vi "DrawOutlines.vi"(8 "BuildingInfoArray":T5(array[cluster])=[{"BuildAverage"={"x"=197.5, "y"=307.5, "z"=77.5}, "BuildIndex"=1, "BuildMax"={"x"=337.0, "y"=500.0, "z"=155.0}, "BuildMin"={"x"=58.0, "y"=115.0, "z"=0.0}}, {"BuildAverage"={"x"=575.0, "y"=290.5, "z"=75.0}, "BuildIndex"=2, "BuildMax"={"x"=712.0, "y"=490.0, "z"=150.0}, "BuildMin"={"x"=438.0, "y"=91.0, "z"=0.0}}, {"BuildAverage"={"x"=-829.0, "y"=-490.5, "z"=36.5}, "BuildIndex"=3, "BuildMax"={"x"=-764.0, "y"=-308.0, "z"=73.0}, "BuildMin"={"x"=-894.0, "y"=-673.0, "z"=0.0}}, {"BuildAverage"={"x"=228.76190476190476, "y"=854.4761904761905, "z"=48.23809523809524}, "BuildIndex"=4, "BuildMax"={"x"=347.0, "y"=1250.0, "z"=108.0}, "BuildMin"={"x"=53.0, "y"=587.0, "z"=0.0}}, {"BuildAverage"={"x"=476.0, "y"=889.25, "z"=51.0}, "BuildIndex"=5, "BuildMax"={"x"=510.0, "y"=1250.0, "z"=102.0}, "BuildMin"={"x"=442.0, "y"=596.0, "z"=0.0}}, {"BuildAverage"={"x"=639.0, "y"=923.0, "z"=68.5}, "BuildIndex"=6, "BuildMax"={"x"=711.0, "y"=1250.0, "z"=137.0}, "BuildMin"={"x"=567.0, "y"=596.0, "z"=0.0}}, {"BuildAverage"={"x"=-264.0, "y"=966.0, "z"=40.0}, "BuildIndex"=7, "BuildMax"={"x"=-43.0, "y"=1043.0, "z"=80.0}, "BuildMin"={"x"=-485.0, "y"=889.0, "z"=0.0}}, {"BuildAverage"={"x"=954.0, "y"=-236.0, "z"=50.0}, "BuildIndex"=8, "BuildMax"={"x"=1086.0, "y"=-130.0, "z"=100.0}, "BuildMin"={"x"=822.0, "y"=-342.0, "z"=0.0}}, {"BuildAverage"={"x"=570.0, "y"=-884.5, "z"=52.0}, "BuildIndex"=9, "BuildMax"={"x"=707.0, "y"=-750.0, "z"=104.0}, "BuildMin"={"x"=433.0, "y"=-1019.0, "z"=0.0}}, {"BuildAverage"={"x"=207.0, "y"=-887.0, "z"=44.0}, "BuildIndex"=10, "BuildMax"={"x"=356.0, "y"=-755.0, "z"=88.0}, "BuildMin"={"x"=58.0, "y"=-1019.0, "z"=0.0}}, {"BuildAverage"={"x"=-154.0, "y"=-887.0, "z"=35.0}, "BuildIndex"=11, "BuildMax"={"x"=-48.0, "y"=-755.0, "z"=70.0}, "BuildMin"={"x"=-260.0, "y"=-1019.0, "z"=0.0}}, {"BuildAverage"={"x"=-380.0, "y"=-887.0, "z"=36.0}, "BuildIndex"=12, "BuildMax"={"x"=-279.0, "y"=-755.0, "z"=72.0}, "BuildMin"={"x"=-481.0, "y"=-1019.0, "z"=0.0}}, {"BuildAverage"={"x"=-1061.2, "y"=-363.6, "z"=46.5}, "BuildIndex"=13, "BuildMax"={"x"=-966.0, "y"=-106.0, "z"=93.0}, "BuildMin"={"x"=-1139.0, "y"=-683.0, "z"=0.0}}, {"BuildAverage"={"x"=-1050.75, "y"=305.0, "z"=84.0}, "BuildIndex"=14, "BuildMax"={"x"=-885.0, "y"=490.0, "z"=168.0}, "BuildMin"={"x"=-1250.0, "y"=120.0, "z"=0.0}}, {"BuildAverage"={"x"=-654.0, "y"=1031.5, "z"=42.5}, "BuildIndex"=15, "BuildMax"={"x"=-577.0, "y"=1481.0, "z"=85.0}, "BuildMin"={"x"=-731.0, "y"=582.0, "z"=0.0}}, {"BuildAverage"={"x"=969.0, "y"=-711.5, "z"=37.5}, "BuildIndex"=16, "BuildMax"={"x"=1106.0, "y"=-404.0, "z"=75.0}, "BuildMin"={"x"=832.0, "y"=-1019.0, "z"=0.0}}, {"BuildAverage"={"x"=1139.5, "y"=425.75, "z"=79.5}, "BuildIndex"=17, "BuildMax"={"x"=1452.0, "y"=1058.0, "z"=159.0}, "BuildMin"={"x"=827.0, "y"=130.0, "z"=0.0}}, {"BuildAverage"={"x"=-1017.6666666666666, "y"=1054.3333333333333, "z"=39.0}, "BuildIndex"=18, "BuildMax"={"x"=-774.0, "y"=1635.0, "z"=78.0}, "BuildMin"={"x"=-1337.0, "y"=663.0, "z"=0.0}}, {"BuildAverage"={"x"=1262.25, "y"=-572.0, "z"=52.5}, "BuildIndex"=19, "BuildMax"={"x"=1404.0, "y"=-125.0, "z"=105.0}, "BuildMin"={"x"=1183.0, "y"=-1019.0, "z"=0.0}}, {"BuildAverage"={"x"=1596.5, "y"=-168.0, "z"=60.0}, "BuildIndex"=20, "BuildMax"={"x"=1885.0, "y"=-115.0, "z"=120.0}, "BuildMin"={"x"=1308.0, "y"=-221.0, "z"=0.0}}, {"BuildAverage"={"x"=1425.0, "y"=-392.0, "z"=50.0}, "BuildIndex"=21, "BuildMax"={"x"=1461.0, "y"=-274.0, "z"=100.0}, "BuildMin"={"x"=1389.0, "y"=-510.0, "z"=0.0}}, {"BuildAverage"={"x"=1577.0, "y"=-479.0, "z"=160.0}, "BuildIndex"=22, "BuildMax"={"x"=1625.0, "y"=-438.0, "z"=320.0}, "BuildMin"={"x"=1529.0, "y"=-520.0, "z"=0.0}}, {"BuildAverage"={"x"=1577.0, "y"=-608.0, "z"=160.0}, "BuildIndex"=23, "BuildMax"={"x"=1625.0, "y"=-543.0, "z"=320.0}, "BuildMin"={"x"=1529.0, "y"=-673.0, "z"=0.0}}, {"BuildAverage"={"x"=1705.75, "y"=-342.75, "z"=37.5}, "BuildIndex"=24, "BuildMax"={"x"=1803.0, "y"=-255.0, "z"=75.0}, "BuildMin"={"x"=1558.0, "y"=-423.0, "z"=0.0}}, {"BuildAverage"={"x"=1790.167058823529, "y"=186.08470588235298, "z"=42.23529411764706}, "BuildIndex"=25, "BuildMax"={"x"=2375.0, "y"=307.69, "z"=95.0}, "BuildMin"={"x"=1548.1, "y"=86.54, "z"=0.0}}, {"BuildAverage"={"x"=-1037.0499999999997, "y"=-832.2999999999997, "z"=33.75}, "BuildIndex"=26, "BuildMax"={"x"=-949.55, "y"=-754.8, "z"=67.5}, "BuildMin"={"x"=-1139.55, "y"=-864.8, "z"=0.0}}, {"BuildAverage"={"x"=-1262.0499999999997, "y"=-923.5333333333334, "z"=35.0}, "BuildIndex"=27, "BuildMax"={"x"=-1097.05, "y"=-769.2, "z"=70.0}, "BuildMin"={"x"=-1492.05, "y"=-1039.2, "z"=0.0}}, {"BuildAverage"={"x"=-160.5, "y"=-1294.95, "z"=45.0}, "BuildIndex"=28, "BuildMax"={"x"=-53.0, "y"=-1099.95, "z"=90.0}, "BuildMin"={"x"=-268.0, "y"=-1489.95, "z"=0.0}}, {"BuildAverage"={"x"=-384.25, "y"=-1294.95, "z"=43.75}, "BuildIndex"=29, "BuildMax"={"x"=-284.25, "y"=-1099.95, "z"=87.5}, "BuildMin"={"x"=-484.25, "y"=-1489.95, "z"=0.0}}, {"BuildAverage"={"x"=-789.25, "y"=-1288.0, "z"=45.0}, "BuildIndex"=30, "BuildMax"={"x"=-576.75, "y"=-1098.0, "z"=90.0}, "BuildMin"={"x"=-1001.75, "y"=-1478.0, "z"=0.0}}, {"BuildAverage"={"x"=-1293.2, "y"=-1283.0, "z"=50.0}, "BuildIndex"=31, "BuildMax"={"x"=-1098.2, "y"=-1098.0, "z"=100.0}, "BuildMin"={"x"=-1488.2, "y"=-1468.0, "z"=0.0}}, {"BuildAverage"={"x"=-940.8500000000001, "y"=-979.9799999999998, "z"=35.0}, "BuildIndex"=32, "BuildMax"={"x"=-884.6, "y"=-940.73, "z"=70.0}, "BuildMin"={"x"=-997.1, "y"=-1019.23, "z"=0.0}}, {"BuildAverage"={"x"=-743.1111111111111, "y"=-891.7777777777778, "z"=31.11111111111111}, "BuildIndex"=33, "BuildMax"={"x"=-567.0, "y"=-755.0, "z"=70.0}, "BuildMin"={"x"=-884.0, "y"=-1019.0, "z"=0.0}}, {"BuildAverage"={"x"=133.0, "y"=-1294.95, "z"=38.75}, "BuildIndex"=34, "BuildMax"={"x"=213.0, "y"=-1099.95, "z"=77.5}, "BuildMin"={"x"=53.0, "y"=-1489.95, "z"=0.0}}, {"BuildAverage"={"x"=298.05, "y"=-1294.95, "z"=42.5}, "BuildIndex"=35, "BuildMax"={"x"=360.55, "y"=-1099.95, "z"=85.0}, "BuildMin"={"x"=235.55, "y"=-1489.95, "z"=0.0}}, {"BuildAverage"={"x"=568.25, "y"=-1294.95, "z"=41.25}, "BuildIndex"=36, "BuildMax"={"x"=718.25, "y"=-1099.95, "z"=82.5}, "BuildMin"={"x"=418.25, "y"=-1489.95, "z"=0.0}}, {"BuildAverage"={"x"=899.3999999999999, "y"=-1294.95, "z"=50.0}, "BuildIndex"=37, "BuildMax"={"x"=971.9, "y"=-1099.95, "z"=100.0}, "BuildMin"={"x"=826.9, "y"=-1489.95, "z"=0.0}}, {"BuildAverage"={"x"=1061.25, "y"=-1294.95, "z"=35.0}, "BuildIndex"=38, "BuildMax"={"x"=1130.0, "y"=-1099.95, "z"=70.0}, "BuildMin"={"x"=1000.0, "y"=-1489.95, "z"=0.0}}, {"BuildAverage"={"x"=-264.0, "y"=389.5, "z"=44.0}, "BuildIndex"=39, "BuildMax"={"x"=-38.0, "y"=500.0, "z"=88.0}, "BuildMin"={"x"=-490.0, "y"=279.0, "z"=0.0}}, {"BuildAverage"={"x"=-418.5, "y"=-226.5, "z"=37.5}, "BuildIndex"=40, "BuildMax"={"x"=-361.0, "y"=-135.0, "z"=75.0}, "BuildMin"={"x"=-476.0, "y"=-318.0, "z"=0.0}}, {"BuildAverage"={"x"=-185.5, "y"=-221.5, "z"=158.5}, "BuildIndex"=41, "BuildMax"={"x"=-58.0, "y"=-135.0, "z"=245.0}, "BuildMin"={"x"=-313.0, "y"=-308.0, "z"=0.0}}, {"BuildAverage"={"x"=394.0, "y"=-224.0, "z"=57.5}, "BuildIndex"=42, "BuildMax"={"x"=721.0, "y"=-130.0, "z"=115.0}, "BuildMin"={"x"=67.0, "y"=-318.0, "z"=0.0}}, {"BuildAverage"={"x"=-387.0, "y"=-519.5, "z"=34.0}, "BuildIndex"=43, "BuildMax"={"x"=-293.0, "y"=-356.0, "z"=68.0}, "BuildMin"={"x"=-481.0, "y"=-683.0, "z"=0.0}}, {"BuildAverage"={"x"=-154.0, "y"=-514.5, "z"=45.0}, "BuildIndex"=44, "BuildMax"={"x"=-48.0, "y"=-356.0, "z"=90.0}, "BuildMin"={"x"=-260.0, "y"=-673.0, "z"=0.0}}, {"BuildAverage"={"x"=370.5, "y"=-513.5, "z"=42.0}, "BuildIndex"=45, "BuildMax"={"x"=712.0, "y"=-404.0, "z"=84.0}, "BuildMin"={"x"=58.0, "y"=-668.0, "z"=0.0}}, {"BuildAverage"={"x"=353.5, "y"=-464.0, "z"=60.0}, "BuildIndex"=46, "BuildMax"={"x"=534.0, "y"=-404.0, "z"=120.0}, "BuildMin"={"x"=173.0, "y"=-524.0, "z"=0.0}}, {"BuildAverage"={"x"=-634.5, "y"=-394.0, "z"=60.0}, "BuildIndex"=47, "BuildMax"={"x"=-567.0, "y"=-115.0, "z"=120.0}, "BuildMin"={"x"=-702.0, "y"=-673.0, "z"=0.0}}, {"BuildAverage"={"x"=-675.5, "y"=288.5, "z"=64.0}, "BuildIndex"=48, "BuildMax"={"x"=-572.0, "y"=495.0, "z"=128.0}, "BuildMin"={"x"=-779.0, "y"=82.0, "z"=0.0}}, {"BuildAverage"={"x"=-829.5, "y"=-197.5, "z"=62.5}, "BuildIndex"=49, "BuildMax"={"x"=-760.0, "y"=-106.0, "z"=125.0}, "BuildMin"={"x"=-899.0, "y"=-289.0, "z"=0.0}}, {"BuildAverage"={"x"=-269.25, "y"=690.0, "z"=0.0}, "BuildIndex"=50, "BuildMax"={"x"=-38.0, "y"=798.0, "z"=0.0}, "BuildMin"={"x"=-500.0, "y"=587.0, "z"=0.0}}, {"BuildAverage"={"x"=-317.25, "y"=168.5, "z"=93.75}, "BuildIndex"=51, "BuildMax"={"x"=-48.0, "y"=250.0, "z"=265.0}, "BuildMin"={"x"=-490.0, "y"=87.0, "z"=0.0}}], 11 "FloorplanArray":T6(array[cluster])=[{"xVert"=337.0, "yVert"=115.0, "zVert"=30.0, "xNorm"=0.0, "yNorm"=0.0, "zNorm"=-1.0, "BuildIndex"=1}, {"xVert"=337.0, "yVert"=115.0, "zVert"=0.0, "xNorm"=0.0, "yNorm"=0.0, "zNorm"=-1.0, "BuildIndex"=1}, {"xVert"=58.0, "yVert"=115.0, "zVert"=0.0, "xNorm"=0.0, "yNorm"=0.0, "zNorm"=-1.0, "BuildIndex"=1}, {"xVert"=58.0, "yVert"=500.0, "zVert"=0.0, "xNorm"=0.0, "yNorm"=0.0, "zNorm"=-1.0, "BuildIndex"=1}, {"xVert"=337.0, "yVert"=500.0, "zVert"=0.0, "xNorm"=0.0, "yNorm"=0.0, "zNorm"=-1.0, "BuildIndex"=1}, {"xVert"=337.0, "yVert"=115.0, "zVert"=0.0, "xNorm"=0.0, "yNorm"=0.0, "zNorm"=-1.0, "BuildIndex"=1}, {"xVert"=337.0, "yVert"=115.0, "zVert"=30.0, "xNorm"=0.0, "yNorm"=0.0, "zNorm"=-1.0, "BuildIndex"=1}, {"xVert"=712.0, "yVert"=91.0, "zVert"=30.0, "xNorm"=0.0, "yNorm"=0.0, "zNorm"=-1.0, "BuildIndex"=2}, {"xVert"=712.0, "yVert"=91.0, "zVert"=0.0, "xNorm"=0.0, "yNorm"=0.0, "zNorm"=-1.0, "BuildIndex"=2}, {"xVert"=438.0, "yVert"=91.0, "zVert"=0.0, "xNorm"=0.0, "yNorm"=0.0, "zNorm"=-1.0, "BuildIndex"=2}, {"xVert"=438.0, "yVert"=490.0, "zVert"=0.0, "xNorm"=0.0, "yNorm"=0.0, "zNorm"=-1.0, "BuildIndex"=2}, {"xVert"=712.0, "yVert"=490.0, "zVert"=0.0, "xNorm"=0.0, "yNorm"=0.0, "zNorm"=-1.0, "BuildIndex"=2}, {"xVert"=712.0, "yVert"=91.0, "zVert"=0.0, "xNorm"=0.0, "yNorm"=0.0, "zNorm"=-1.0, "BuildIndex"=2}, {"xVert"=712.0, "yVert"=91.0, "zVert"=30.0, "xNorm"=0.0, "yNorm"=0.0, "zNorm"=-1.0, "BuildIndex"=2}, {"xVert"=-764.0, "yVert"=-308.0, "zVert"=30.0, "xNorm"=0.0, "yNorm"=0.0, "zNorm"=-1.0, "BuildIndex"=3}, {"xVert"=-764.0, "yVert"=-308.0, "zVert"=0.0, "xNorm"=0.0, "yNorm"=0.0, "zNorm"=-1.0, "BuildIndex"=3}, {"xVert"=-764.0, "yVert"=-673.0, "zVert"=0.0, "xNorm"=0.0, "yNorm"=0.0, "zNorm"=-1.0, "BuildIndex"=3}, {"xVert"=-894.0, "yVert"=-673.0, "zVert"=0.0, "xNorm"=0.0, "yNorm"=0.0, "zNorm"=-1.0, "BuildIndex"=3}, {"xVert"=-894.0, "yVert"=-308.0, "zVert"=0.0, "xNorm"=0.0, "yNorm"=0.0, "zNorm"=-1.0, "BuildIndex"=3}, {"xVert"=-764.0, "yVert"=-308.0, "zVert"=0.0, "xNorm"=0.0, "yNorm"=0.0, "zNorm"=-1.0, "BuildIndex"=3}, {"xVert"=-764.0, "yVert"=-308.0, "zVert"=30.0, "xNorm"=0.0, "yNorm"=0.0, "zNorm"=-1.0, "BuildIndex"=3}, {"xVert"=53.0, "yVert"=587.0, "zVert"=30.0, "xNorm"=0.0, "yNorm"=0.0, "zNorm"=-1.0, "BuildIndex"=4}, {"xVert"=53.0, "yVert"=587.0, "zVert"=0.0, "xNorm"=0.0, "yNorm"=0.0, "zNorm"=-1.0, "BuildIndex"=4}, {"xVert"=53.0, "yVert"=1250.0, "zVert"=0.0, "xNorm"=0.0, "yNorm"=0.0, "zNorm"=-1.0, "BuildIndex"=4}, {"xVert"=216.0, "yVert"=1250.0, "zVert"=0.0, "xNorm"=0.0, "yNorm"=0.0, "zNorm"=-1.0, "BuildIndex"=4}, {"xVert"=216.0, "yVert"=654.0, "zVert"=0.0, "xNorm"=0.0, "yNorm"=0.0, "zNorm"=-1.0, "BuildIndex"=4}, {"xVert"=260.0, "yVert"=654.0, "zVert"=0.0, "xNorm"=0.0, "yNorm"=0.0, "zNorm"=-1.0, "BuildIndex"=4}, {"xVert"=260.0, "yVert"=596.0, "zVert"=0.0, "xNorm"=0.0, "yNorm"=0.0, "zNorm"=-1.0, "BuildIndex"=4}, {"xVert"=260.0, "yVert"=587.0, "zVert"=0.0, "xNorm"=0.0, "yNorm"=0.0, "zNorm"=-1.0, "BuildIndex"=4}, {"xVert"=260.0, "yVert"=596.0, "zVert"=0.0, "xNorm"=0.0, "yNorm"=0.0, "zNorm"=-1.0, "BuildIndex"=4}, {"xVert"=260.0, "yVert"=654.0, "zVert"=0.0, "xNorm"=0.0, "yNorm"=0.0, "zNorm"=-1.0, "BuildIndex"=4}, {"xVert"=260.0, "yVert"=1250.0, "zVert"=0.0, "xNorm"=0.0, "yNorm"=0.0, "zNorm"=-1.0, "BuildIndex"=4}, {"xVert"=347.0, "yVert"=1250.0, "zVert"=0.0, "xNorm"=0.0, "yNorm"=0.0, "zNorm"=-1.0, "BuildIndex"=4}, {"xVert"=347.0, "yVert"=596.0, "zVert"=0.0, "xNorm"=0.0, "yNorm"=0.0, "zNorm"=-1.0, "BuildIndex"=4}, {"xVert"=53.0, "yVert"=587.0, "zVert"=0.0, "xNorm"=0.0, "yNorm"=0.0, "zNorm"=-1.0, "BuildIndex"=4}, {"xVert"=53.0, "yVert"=587.0, "zVert"=30.0, "xNorm"=0.0, "yNorm"=0.0, "zNorm"=-1.0, "BuildIndex"=4}, {"xVert"=442.0, "yVert"=596.0, "zVert"=30.0, "xNorm"=0.0, "yNorm"=0.0, "zNorm"=-1.0, "BuildIndex"=5}, {"xVert"=442.0, "yVert"=596.0, "zVert"=0.0, "xNorm"=0.0, "yNorm"=0.0, "zNorm"=-1.0, "BuildIndex"=5}, {"xVert"=442.0, "yVert"=1250.0, "zVert"=0.0, "xNorm"=0.0, "yNorm"=0.0, "zNorm"=-1.0, "BuildIndex"=5}, {"xVert"=510.0, "yVert"=1115.0, "zVert"=0.0, "xNorm"=0.0, "yNorm"=0.0, "zNorm"=-1.0, "BuildIndex"=5}, {"xVert"=510.0, "yVert"=596.0, "zVert"=0.0, "xNorm"=0.0, "yNorm"=0.0, "zNorm"=-1.0, "BuildIndex"=5}, {"xVert"=442.0, "yVert"=596.0, "zVert"=0.0, "xNorm"=0.0, "yNorm"=0.0, "zNorm"=-1.0, "BuildIndex"=5}, {"xVert"=442.0, "yVert"=596.0, "zVert"=30.0, "xNorm"=0.0, "yNorm"=0.0, "zNorm"=-1.0, "BuildIndex"=5}, {"xVert"=711.0, "yVert"=596.0, "zVert"=30.0, "xNorm"=0.0, "yNorm"=0.0, "zNorm"=-1.0, "BuildIndex"=6}, {"xVert"=711.0, "yVert"=596.0, "zVert"=0.0, "xNorm"=0.0, "yNorm"=0.0, "zNorm"=-1.0, "BuildIndex"=6}, {"xVert"=567.0, "yVert"=596.0, "zVert"=0.0, "xNorm"=0.0, "yNorm"=0.0, "zNorm"=-1.0, "BuildIndex"=6}, {"xVert"=567.0, "yVert"=1250.0, "zVert"=0.0, "xNorm"=0.0, "yNorm"=0.0, "zNorm"=-1.0, "BuildIndex"=6}, {"xVert"=711.0, "yVert"=1250.0, "zVert"=0.0, "xNorm"=0.0, "yNorm"=0.0, "zNorm"=-1.0, "BuildIndex"=6}, {"xVert"=711.0, "yVert"=596.0, "zVert"=0.0, "xNorm"=0.0, "yNorm"=0.0, "zNorm"=-1.0, "BuildIndex"=6}, {"xVert"=711.0, "yVert"=596.0, "zVert"=30.0, "xNorm"=0.0, "yNorm"=0.0, "zNorm"=-1.0, "BuildIndex"=6}, {"xVert"=-43.0, "yVert"=889.0, "zVert"=30.0, "xNorm"=0.0, "yNorm"=0.0, "zNorm"=-1.0, "BuildIndex"=7}, {"xVert"=-43.0, "yVert"=889.0, "zVert"=0.0, "xNorm"=0.0, "yNorm"=0.0, "zNorm"=-1.0, "BuildIndex"=7}, {"xVert"=-485.0, "yVert"=889.0, "zVert"=0.0, "xNorm"=0.0, "yNorm"=0.0, "zNorm"=-1.0, "BuildIndex"=7}, {"xVert"=-485.0, "yVert"=1043.0, "zVert"=0.0, "xNorm"=0.0, "yNorm"=0.0, "zNorm"=-1.0, "BuildIndex"=7}, {"xVert"=-43.0, "yVert"=1043.0, "zVert"=0.0, "xNorm"=0.0, "yNorm"=0.0, "zNorm"=-1.0, "BuildIndex"=7}, {"xVert"=-43.0, "yVert"=889.0, "zVert"=0.0, "xNorm"=0.0, "yNorm"=0.0, "zNorm"=-1.0, "BuildIndex"=7}, {"xVert"=-43.0, "yVert"=889.0, "zVert"=30.0, "xNorm"=0.0, "yNorm"=0.0, "zNorm"=-1.0, "BuildIndex"=7}, {"xVert"=822.0, "yVert"=-130.0, "zVert"=30.0, "xNorm"=0.0, "yNorm"=0.0, "zNorm"=-1.0, "BuildIndex"=8}, {"xVert"=822.0, "yVert"=-130.0, "zVert"=0.0, "xNorm"=0.0, "yNorm"=0.0, "zNorm"=-1.0, "BuildIndex"=8}, {"xVert"=1086.0, "yVert"=-130.0, "zVert"=0.0, "xNorm"=0.0, "yNorm"=0.0, "zNorm"=-1.0, "BuildIndex"=8}, {"xVert"=1086.0, "yVert"=-342.0, "zVert"=0.0, "xNorm"=0.0, "yNorm"=0.0, "zNorm"=-1.0, "BuildIndex"=8}, {"xVert"=822.0, "yVert"=-342.0, "zVert"=0.0, "xNorm"=0.0, "yNorm"=0.0, "zNorm"=-1.0, "BuildIndex"=8}, {"xVert"=822.0, "yVert"=-130.0, "zVert"=0.0, "xNorm"=0.0, "yNorm"=0.0, "zNorm"=-1.0, "BuildIndex"=8}, {"xVert"=822.0, "yVert"=-130.0, "zVert"=30.0, "xNorm"=0.0, "yNorm"=0.0, "zNorm"=-1.0, "BuildIndex"=8}, {"xVert"=433.0, "yVert"=-750.0, "zVert"=30.0, "xNorm"=0.0, "yNorm"=0.0, "zNorm"=-1.0, "BuildIndex"=9}, {"xVert"=433.0, "yVert"=-750.0, "zVert"=0.0, "xNorm"=0.0, "yNorm"=0.0, "zNorm"=-1.0, "BuildIndex"=9}, {"xVert"=707.0, "yVert"=-750.0, "zVert"=0.0, "xNorm"=0.0, "yNorm"=0.0, "zNorm"=-1.0, "BuildIndex"=9}, {"xVert"=707.0, "yVert"=-1019.0, "zVert"=0.0, "xNorm"=0.0, "yNorm"=0.0, "zNorm"=-1.0, "BuildIndex"=9}, {"xVert"=433.0, "yVert"=-1019.0, "zVert"=0.0, "xNorm"=0.0, "yNorm"=0.0, "zNorm"=-1.0, "BuildIndex"=9}, {"xVert"=433.0, "yVert"=-750.0, "zVert"=0.0, "xNorm"=0.0, "yNorm"=0.0, "zNorm"=-1.0, "BuildIndex"=9}, {"xVert"=433.0, "yVert"=-750.0, "zVert"=30.0, "xNorm"=0.0, "yNorm"=0.0, "zNorm"=-1.0, "BuildIndex"=9}, {"xVert"=58.0, "yVert"=-755.0, "zVert"=30.0, "xNorm"=0.0, "yNorm"=0.0, "zNorm"=-1.0, "BuildIndex"=10}, {"xVert"=58.0, "yVert"=-755.0, "zVert"=0.0, "xNorm"=0.0, "yNorm"=0.0, "zNorm"=-1.0, "BuildIndex"=10}, {"xVert"=356.0, "yVert"=-755.0, "zVert"=0.0, "xNorm"=0.0, "yNorm"=0.0, "zNorm"=-1.0, "BuildIndex"=10}, {"xVert"=356.0, "yVert"=-1019.0, "zVert"=0.0, "xNorm"=0.0, "yNorm"=0.0, "zNorm"=-1.0, "BuildIndex"=10}, {"xVert"=58.0, "yVert"=-1019.0, "zVert"=0.0, "xNorm"=0.0, "yNorm"=0.0, "zNorm"=-1.0, "BuildIndex"=10}, {"xVert"=58.0, "yVert"=-755.0, "zVert"=0.0, "xNorm"=0.0, "yNorm"=0.0, "zNorm"=-1.0, "BuildIndex"=10}, {"xVert"=58.0, "yVert"=-755.0, "zVert"=30.0, "xNorm"=0.0, "yNorm"=0.0, "zNorm"=-1.0, "BuildIndex"=10}, {"xVert"=-260.0, "yVert"=-755.0, "zVert"=30.0, "xNorm"=0.0, "yNorm"=0.0, "zNorm"=-1.0, "BuildIndex"=11}, {"xVert"=-260.0, "yVert"=-755.0, "zVert"=0.0, "xNorm"=0.0, "yNorm"=0.0, "zNorm"=-1.0, "BuildIndex"=11}, {"xVert"=-48.0, "yVert"=-755.0, "zVert"=0.0, "xNorm"=0.0, "yNorm"=0.0, "zNorm"=-1.0, "BuildIndex"=11}, {"xVert"=-48.0, "yVert"=-1019.0, "zVert"=0.0, "xNorm"=0.0, "yNorm"=0.0, "zNorm"=-1.0, "BuildIndex"=11}, {"xVert"=-260.0, "yVert"=-1019.0, "zVert"=0.0, "xNorm"=0.0, "yNorm"=0.0, "zNorm"=-1.0, "BuildIndex"=11}, {"xVert"=-260.0, "yVert"=-755.0, "zVert"=0.0, "xNorm"=0.0, "yNorm"=0.0, "zNorm"=-1.0, "BuildIndex"=11}, {"xVert"=-260.0, "yVert"=-755.0, "zVert"=30.0, "xNorm"=0.0, "yNorm"=0.0, "zNorm"=-1.0, "BuildIndex"=11}, {"xVert"=-481.0, "yVert"=-755.0, "zVert"=30.0, "xNorm"=0.0, "yNorm"=0.0, "zNorm"=-1.0, "BuildIndex"=12}, {"xVert"=-481.0, "yVert"=-755.0, "zVert"=0.0, "xNorm"=0.0, "yNorm"=0.0, "zNorm"=-1.0, "BuildIndex"=12}, {"xVert"=-279.0, "yVert"=-755.0, "zVert"=0.0, "xNorm"=0.0, "yNorm"=0.0, "zNorm"=-1.0, "BuildIndex"=12}, {"xVert"=-279.0, "yVert"=-1019.0, "zVert"=0.0, "xNorm"=0.0, "yNorm"=0.0, "zNorm"=-1.0, "BuildIndex"=12}, {"xVert"=-481.0, "yVert"=-1019.0, "zVert"=0.0, "xNorm"=0.0, "yNorm"=0.0, "zNorm"=-1.0, "BuildIndex"=12}, {"xVert"=-481.0, "yVert"=-755.0, "zVert"=0.0, "xNorm"=0.0, "yNorm"=0.0, "zNorm"=-1.0, "BuildIndex"=12}, {"xVert"=-481.0, "yVert"=-755.0, "zVert"=30.0, "xNorm"=0.0, "yNorm"=0.0, "zNorm"=-1.0, "BuildIndex"=12}, {"xVert"=-1139.0, "yVert"=-240.0, "zVert"=30.0, "xNorm"=0.0, "yNorm"=0.0, "zNorm"=-1.0, "BuildIndex"=13}, {"xVert"=-1139.0, "yVert"=-240.0, "zVert"=0.0, "xNorm"=0.0, "yNorm"=0.0, "zNorm"=-1.0, "BuildIndex"=13}, {"xVert"=-1139.0, "yVert"=-106.0, "zVert"=0.0, "xNorm"=0.0, "yNorm"=0.0, "zNorm"=-1.0, "BuildIndex"=13}, {"xVert"=-966.0, "yVert"=-106.0, "zVert"=0.0, "xNorm"=0.0, "yNorm"=0.0, "zNorm"=-1.0, "BuildIndex"=13}, {"xVert"=-966.0, "yVert"=-683.0, "zVert"=0.0, "xNorm"=0.0, "yNorm"=0.0, "zNorm"=-1.0, "BuildIndex"=13}, {"xVert"=-1096.0, "yVert"=-683.0, "zVert"=0.0, "xNorm"=0.0, "yNorm"=0.0, "zNorm"=-1.0, "BuildIndex"=13}, {"xVert"=-1139.0, "yVert"=-240.0, "zVert"=0.0, "xNorm"=0.0, "yNorm"=0.0, "zNorm"=-1.0, "BuildIndex"=13}, {"xVert"=-1139.0, "yVert"=-240.0, "zVert"=30.0, "xNorm"=0.0, "yNorm"=0.0, "zNorm"=-1.0, "BuildIndex"=13}, {"xVert"=-885.0, "yVert"=490.0, "zVert"=30.0, "xNorm"=0.0, "yNorm"=0.0, "zNorm"=-1.0, "BuildIndex"=14}, {"xVert"=-885.0, "yVert"=490.0, "zVert"=0.0, "xNorm"=0.0, "yNorm"=0.0, "zNorm"=-1.0, "BuildIndex"=14}, {"xVert"=-885.0, "yVert"=120.0, "zVert"=0.0, "xNorm"=0.0, "yNorm"=0.0, "zNorm"=-1.0, "BuildIndex"=14}, {"xVert"=-1183.0, "yVert"=120.0, "zVert"=0.0, "xNorm"=0.0, "yNorm"=0.0, "zNorm"=-1.0, "BuildIndex"=14}, {"xVert"=-1250.0, "yVert"=490.0, "zVert"=0.0, "xNorm"=0.0, "yNorm"=0.0, "zNorm"=-1.0, "BuildIndex"=14}, {"xVert"=-885.0, "yVert"=490.0, "zVert"=0.0, "xNorm"=0.0, "yNorm"=0.0, "zNorm"=-1.0, "BuildIndex"=14}, {"xVert"=-885.0, "yVert"=490.0, "zVert"=30.0, "xNorm"=0.0, "yNorm"=0.0, "zNorm"=-1.0, "BuildIndex"=14}, {"xVert"=-577.0, "yVert"=1481.0, "zVert"=30.0, "xNorm"=0.0, "yNorm"=0.0, "zNorm"=-1.0, "BuildIndex"=15}, {"xVert"=-577.0, "yVert"=1481.0, "zVert"=0.0, "xNorm"=0.0, "yNorm"=0.0, "zNorm"=-1.0, "BuildIndex"=15}, {"xVert"=-577.0, "yVert"=582.0, "zVert"=0.0, "xNorm"=0.0, "yNorm"=0.0, "zNorm"=-1.0, "BuildIndex"=15}, {"xVert"=-731.0, "yVert"=582.0, "zVert"=0.0, "xNorm"=0.0, "yNorm"=0.0, "zNorm"=-1.0, "BuildIndex"=15}, {"xVert"=-731.0, "yVert"=1481.0, "zVert"=0.0, "xNorm"=0.0, "yNorm"=0.0, "zNorm"=-1.0, "BuildIndex"=15}, {"xVert"=-577.0, "yVert"=1481.0, "zVert"=0.0, "xNorm"=0.0, "yNorm"=0.0, "zNorm"=-1.0, "BuildIndex"=15}, {"xVert"=-577.0, "yVert"=1481.0, "zVert"=30.0, "xNorm"=0.0, "yNorm"=0.0, "zNorm"=-1.0, "BuildIndex"=15}, {"xVert"=832.0, "yVert"=-404.0, "zVert"=30.0, "xNorm"=0.0, "yNorm"=0.0, "zNorm"=-1.0, "BuildIndex"=16}, {"xVert"=832.0, "yVert"=-404.0, "zVert"=0.0, "xNorm"=0.0, "yNorm"=0.0, "zNorm"=-1.0, "BuildIndex"=16}, {"xVert"=1106.0, "yVert"=-404.0, "zVert"=0.0, "xNorm"=0.0, "yNorm"=0.0, "zNorm"=-1.0, "BuildIndex"=16}, {"xVert"=1106.0, "yVert"=-1019.0, "zVert"=0.0, "xNorm"=0.0, "yNorm"=0.0, "zNorm"=-1.0, "BuildIndex"=16}, {"xVert"=832.0, "yVert"=-1019.0, "zVert"=0.0, "xNorm"=0.0, "yNorm"=0.0, "zNorm"=-1.0, "BuildIndex"=16}, {"xVert"=832.0, "yVert"=-404.0, "zVert"=0.0, "xNorm"=0.0, "yNorm"=0.0, "zNorm"=-1.0, "BuildIndex"=16}, {"xVert"=832.0, "yVert"=-404.0, "zVert"=30.0, "xNorm"=0.0, "yNorm"=0.0, "zNorm"=-1.0, "BuildIndex"=16}, {"xVert"=1452.0, "yVert"=385.0, "zVert"=30.0, "xNorm"=0.0, "yNorm"=0.0, "zNorm"=-1.0, "BuildIndex"=17}, {"xVert"=1452.0, "yVert"=385.0, "zVert"=0.0, "xNorm"=0.0, "yNorm"=0.0, "zNorm"=-1.0, "BuildIndex"=17}, {"xVert"=1452.0, "yVert"=130.0, "zVert"=0.0, "xNorm"=0.0, "yNorm"=0.0, "zNorm"=-1.0, "BuildIndex"=17}, {"xVert"=827.0, "yVert"=130.0, "zVert"=0.0, "xNorm"=0.0, "yNorm"=0.0, "zNorm"=-1.0, "BuildIndex"=17}, {"xVert"=827.0, "yVert"=1058.0, "zVert"=0.0, "xNorm"=0.0, "yNorm"=0.0, "zNorm"=-1.0, "BuildIndex"=17}, {"xVert"=1452.0, "yVert"=385.0, "zVert"=0.0, "xNorm"=0.0, "yNorm"=0.0, "zNorm"=-1.0, "BuildIndex"=17}, {"xVert"=1452.0, "yVert"=385.0, "zVert"=30.0, "xNorm"=0.0, "yNorm"=0.0, "zNorm"=-1.0, "BuildIndex"=17}, {"xVert"=-1337.0, "yVert"=663.0, "zVert"=30.0, "xNorm"=0.0, "yNorm"=0.0, "zNorm"=-1.0, "BuildIndex"=18}, {"xVert"=-1337.0, "yVert"=663.0, "zVert"=0.0, "xNorm"=0.0, "yNorm"=0.0, "zNorm"=-1.0, "BuildIndex"=18}, {"xVert"=-1337.0, "yVert"=865.0, "zVert"=0.0, "xNorm"=0.0, "yNorm"=0.0, "zNorm"=-1.0, "BuildIndex"=18}, {"xVert"=-942.0, "yVert"=865.0, "zVert"=0.0, "xNorm"=0.0, "yNorm"=0.0, "zNorm"=-1.0, "BuildIndex"=18}, {"xVert"=-942.0, "yVert"=1635.0, "zVert"=0.0, "xNorm"=0.0, "yNorm"=0.0, "zNorm"=-1.0, "BuildIndex"=18}, {"xVert"=-774.0, "yVert"=1635.0, "zVert"=0.0, "xNorm"=0.0, "yNorm"=0.0, "zNorm"=-1.0, "BuildIndex"=18}, {"xVert"=-774.0, "yVert"=663.0, "zVert"=0.0, "xNorm"=0.0, "yNorm"=0.0, "zNorm"=-1.0, "BuildIndex"=18}, {"xVert"=-1337.0, "yVert"=663.0, "zVert"=0.0, "xNorm"=0.0, "yNorm"=0.0, "zNorm"=-1.0, "BuildIndex"=18}, {"xVert"=-1337.0, "yVert"=663.0, "zVert"=30.0, "xNorm"=0.0, "yNorm"=0.0, "zNorm"=-1.0, "BuildIndex"=18}, {"xVert"=1183.0, "yVert"=-1019.0, "zVert"=30.0, "xNorm"=0.0, "yNorm"=0.0, "zNorm"=-1.0, "BuildIndex"=19}, {"xVert"=1183.0, "yVert"=-1019.0, "zVert"=0.0, "xNorm"=0.0, "yNorm"=0.0, "zNorm"=-1.0, "BuildIndex"=19}, {"xVert"=1183.0, "yVert"=-125.0, "zVert"=0.0, "xNorm"=0.0, "yNorm"=0.0, "zNorm"=-1.0, "BuildIndex"=19}, {"xVert"=1279.0, "yVert"=-125.0, "zVert"=0.0, "xNorm"=0.0, "yNorm"=0.0, "zNorm"=-1.0, "BuildIndex"=19}, {"xVert"=1404.0, "yVert"=-1019.0, "zVert"=0.0, "xNorm"=0.0, "yNorm"=0.0, "zNorm"=-1.0, "BuildIndex"=19}, {"xVert"=1183.0, "yVert"=-1019.0, "zVert"=0.0, "xNorm"=0.0, "yNorm"=0.0, "zNorm"=-1.0, "BuildIndex"=19}, {"xVert"=1183.0, "yVert"=-1019.0, "zVert"=30.0, "xNorm"=0.0, "yNorm"=0.0, "zNorm"=-1.0, "BuildIndex"=19}, {"xVert"=1308.0, "yVert"=-115.0, "zVert"=30.0, "xNorm"=0.0, "yNorm"=0.0, "zNorm"=-1.0, "BuildIndex"=20}, {"xVert"=1308.0, "yVert"=-115.0, "zVert"=0.0, "xNorm"=0.0, "yNorm"=0.0, "zNorm"=-1.0, "BuildIndex"=20}, {"xVert"=1885.0, "yVert"=-115.0, "zVert"=0.0, "xNorm"=0.0, "yNorm"=0.0, "zNorm"=-1.0, "BuildIndex"=20}, {"xVert"=1885.0, "yVert"=-221.0, "zVert"=0.0, "xNorm"=0.0, "yNorm"=0.0, "zNorm"=-1.0, "BuildIndex"=20}, {"xVert"=1308.0, "yVert"=-221.0, "zVert"=0.0, "xNorm"=0.0, "yNorm"=0.0, "zNorm"=-1.0, "BuildIndex"=20}, {"xVert"=1308.0, "yVert"=-115.0, "zVert"=0.0, "xNorm"=0.0, "yNorm"=0.0, "zNorm"=-1.0, "BuildIndex"=20}, {"xVert"=1308.0, "yVert"=-115.0, "zVert"=30.0, "xNorm"=0.0, "yNorm"=0.0, "zNorm"=-1.0, "BuildIndex"=20}, {"xVert"=1389.0, "yVert"=-510.0, "zVert"=30.0, "xNorm"=0.0, "yNorm"=0.0, "zNorm"=-1.0, "BuildIndex"=21}, {"xVert"=1389.0, "yVert"=-510.0, "zVert"=0.0, "xNorm"=0.0, "yNorm"=0.0, "zNorm"=-1.0, "BuildIndex"=21}, {"xVert"=1389.0, "yVert"=-274.0, "zVert"=0.0, "xNorm"=0.0, "yNorm"=0.0, "zNorm"=-1.0, "BuildIndex"=21}, {"xVert"=1461.0, "yVert"=-274.0, "zVert"=0.0, "xNorm"=0.0, "yNorm"=0.0, "zNorm"=-1.0, "BuildIndex"=21}, {"xVert"=1461.0, "yVert"=-510.0, "zVert"=0.0, "xNorm"=0.0, "yNorm"=0.0, "zNorm"=-1.0, "BuildIndex"=21}, {"xVert"=1389.0, "yVert"=-510.0, "zVert"=0.0, "xNorm"=0.0, "yNorm"=0.0, "zNorm"=-1.0, "BuildIndex"=21}, {"xVert"=1389.0, "yVert"=-510.0, "zVert"=30.0, "xNorm"=0.0, "yNorm"=0.0, "zNorm"=-1.0, "BuildIndex"=21}, {"xVert"=1529.0, "yVert"=-438.0, "zVert"=30.0, "xNorm"=0.0, "yNorm"=0.0, "zNorm"=-1.0, "BuildIndex"=22}, {"xVert"=1529.0, "yVert"=-438.0, "zVert"=0.0, "xNorm"=0.0, "yNorm"=0.0, "zNorm"=-1.0, "BuildIndex"=22}, {"xVert"=1625.0, "yVert"=-438.0, "zVert"=0.0, "xNorm"=0.0, "yNorm"=0.0, "zNorm"=-1.0, "BuildIndex"=22}, {"xVert"=1625.0, "yVert"=-520.0, "zVert"=0.0, "xNorm"=0.0, "yNorm"=0.0, "zNorm"=-1.0, "BuildIndex"=22}, {"xVert"=1529.0, "yVert"=-520.0, "zVert"=0.0, "xNorm"=0.0, "yNorm"=0.0, "zNorm"=-1.0, "BuildIndex"=22}, {"xVert"=1529.0, "yVert"=-438.0, "zVert"=0.0, "xNorm"=0.0, "yNorm"=0.0, "zNorm"=-1.0, "BuildIndex"=22}, {"xVert"=1529.0, "yVert"=-438.0, "zVert"=30.0, "xNorm"=0.0, "yNorm"=0.0, "zNorm"=-1.0, "BuildIndex"=22}, {"xVert"=1529.0, "yVert"=-543.0, "zVert"=30.0, "xNorm"=0.0, "yNorm"=0.0, "zNorm"=-1.0, "BuildIndex"=23}, {"xVert"=1529.0, "yVert"=-543.0, "zVert"=0.0, "xNorm"=0.0, "yNorm"=0.0, "zNorm"=-1.0, "BuildIndex"=23}, {"xVert"=1625.0, "yVert"=-543.0, "zVert"=0.0, "xNorm"=0.0, "yNorm"=0.0, "zNorm"=-1.0, "BuildIndex"=23}, {"xVert"=1625.0, "yVert"=-673.0, "zVert"=0.0, "xNorm"=0.0, "yNorm"=0.0, "zNorm"=-1.0, "BuildIndex"=23}, {"xVert"=1529.0, "yVert"=-673.0, "zVert"=0.0, "xNorm"=0.0, "yNorm"=0.0, "zNorm"=-1.0, "BuildIndex"=23}, {"xVert"=1529.0, "yVert"=-543.0, "zVert"=0.0, "xNorm"=0.0, "yNorm"=0.0, "zNorm"=-1.0, "BuildIndex"=23}, {"xVert"=1529.0, "yVert"=-543.0, "zVert"=30.0, "xNorm"=0.0, "yNorm"=0.0, "zNorm"=-1.0, "BuildIndex"=23}, {"xVert"=1731.0, "yVert"=-423.0, "zVert"=30.0, "xNorm"=0.0, "yNorm"=0.0, "zNorm"=-1.0, "BuildIndex"=24}, {"xVert"=1731.0, "yVert"=-423.0, "zVert"=0.0, "xNorm"=0.0, "yNorm"=0.0, "zNorm"=-1.0, "BuildIndex"=24}, {"xVert"=1731.0, "yVert"=-385.0, "zVert"=0.0, "xNorm"=0.0, "yNorm"=0.0, "zNorm"=-1.0, "BuildIndex"=24}, {"xVert"=1558.0, "yVert"=-385.0, "zVert"=0.0, "xNorm"=0.0, "yNorm"=0.0, "zNorm"=-1.0, "BuildIndex"=24}, {"xVert"=1558.0, "yVert"=-308.0, "zVert"=0.0, "xNorm"=0.0, "yNorm"=0.0, "zNorm"=-1.0, "BuildIndex"=24}, {"xVert"=1731.0, "yVert"=-308.0, "zVert"=0.0, "xNorm"=0.0, "yNorm"=0.0, "zNorm"=-1.0, "BuildIndex"=24}, {"xVert"=1731.0, "yVert"=-255.0, "zVert"=0.0, "xNorm"=0.0, "yNorm"=0.0, "zNorm"=-1.0, "BuildIndex"=24}, {"xVert"=1803.0, "yVert"=-255.0, "zVert"=0.0, "xNorm"=0.0, "yNorm"=0.0, "zNorm"=-1.0, "BuildIndex"=24}, {"xVert"=1803.0, "yVert"=-423.0, "zVert"=0.0, "xNorm"=0.0, "yNorm"=0.0, "zNorm"=-1.0, "BuildIndex"=24}, {"xVert"=1731.0, "yVert"=-423.0, "zVert"=0.0, "xNorm"=0.0, "yNorm"=0.0, "zNorm"=-1.0, "BuildIndex"=24}, {"xVert"=1731.0, "yVert"=-423.0, "zVert"=30.0, "xNorm"=0.0, "yNorm"=0.0, "zNorm"=-1.0, "BuildIndex"=24}, {"xVert"=1548.1, "yVert"=221.15, "zVert"=30.0, "xNorm"=0.0, "yNorm"=0.0, "zNorm"=-1.0, "BuildIndex"=25}, {"xVert"=1548.1, "yVert"=221.15, "zVert"=0.0, "xNorm"=0.0, "yNorm"=0.0, "zNorm"=-1.0, "BuildIndex"=25}, {"xVert"=1548.1, "yVert"=307.69, "zVert"=0.0, "xNorm"=0.0, "yNorm"=0.0, "zNorm"=-1.0, "BuildIndex"=25}, {"xVert"=2375.0, "yVert"=307.69, "zVert"=0.0, "xNorm"=0.0, "yNorm"=0.0, "zNorm"=-1.0, "BuildIndex"=25}, {"xVert"=2375.0, "yVert"=86.54, "zVert"=0.0, "xNorm"=0.0, "yNorm"=0.0, "zNorm"=-1.0, "BuildIndex"=25}, {"xVert"=1682.69, "yVert"=86.54, "zVert"=0.0, "xNorm"=0.0, "yNorm"=0.0, "zNorm"=-1.0, "BuildIndex"=25}, {"xVert"=1682.69, "yVert"=221.15, "zVert"=0.0, "xNorm"=0.0, "yNorm"=0.0, "zNorm"=-1.0, "BuildIndex"=25}, {"xVert"=1548.1, "yVert"=86.54, "zVert"=0.0, "xNorm"=0.0, "yNorm"=0.0, "zNorm"=-1.0, "BuildIndex"=25}, {"xVert"=1548.1, "yVert"=221.15, "zVert"=0.0, "xNorm"=0.0, "yNorm"=0.0, "zNorm"=-1.0, "BuildIndex"=25}, {"xVert"=1682.69, "yVert"=221.15, "zVert"=0.0, "xNorm"=0.0, "yNorm"=0.0, "zNorm"=-1.0, "BuildIndex"=25}, {"xVert"=1682.69, "yVert"=86.54, "zVert"=0.0, "xNorm"=0.0, "yNorm"=0.0, "zNorm"=-1.0, "BuildIndex"=25}, {"xVert"=1548.1, "yVert"=221.15, "zVert"=0.0, "xNorm"=0.0, "yNorm"=0.0, "zNorm"=-1.0, "BuildIndex"=25}, {"xVert"=1548.1, "yVert"=221.15, "zVert"=30.0, "xNorm"=0.0, "yNorm"=0.0, "zNorm"=-1.0, "BuildIndex"=25}, {"xVert"=-1139.55, "yVert"=-854.8, "zVert"=30.0, "xNorm"=0.0, "yNorm"=0.0, "zNorm"=-1.0, "BuildIndex"=26}, {"xVert"=-1139.55, "yVert"=-854.8, "zVert"=0.0, "xNorm"=0.0, "yNorm"=0.0, "zNorm"=-1.0, "BuildIndex"=26}, {"xVert"=-1139.55, "yVert"=-754.8, "zVert"=0.0, "xNorm"=0.0, "yNorm"=0.0, "zNorm"=-1.0, "BuildIndex"=26}, {"xVert"=-949.55, "yVert"=-754.8, "zVert"=0.0, "xNorm"=0.0, "yNorm"=0.0, "zNorm"=-1.0, "BuildIndex"=26}, {"xVert"=-949.55, "yVert"=-854.8, "zVert"=0.0, "xNorm"=0.0, "yNorm"=0.0, "zNorm"=-1.0, "BuildIndex"=26}, {"xVert"=-1005.8, "yVert"=-854.8, "zVert"=0.0, "xNorm"=0.0, "yNorm"=0.0, "zNorm"=-1.0, "BuildIndex"=26}, {"xVert"=-1005.8, "yVert"=-864.8, "zVert"=0.0, "xNorm"=0.0, "yNorm"=0.0, "zNorm"=-1.0, "BuildIndex"=26}, {"xVert"=-1053.3, "yVert"=-864.8, "zVert"=0.0, "xNorm"=0.0, "yNorm"=0.0, "zNorm"=-1.0, "BuildIndex"=26}, {"xVert"=-1053.3, "yVert"=-854.8, "zVert"=0.0, "xNorm"=0.0, "yNorm"=0.0, "zNorm"=-1.0, "BuildIndex"=26}, {"xVert"=-1139.55, "yVert"=-854.8, "zVert"=0.0, "xNorm"=0.0, "yNorm"=0.0, "zNorm"=-1.0, "BuildIndex"=26}, {"xVert"=-1139.55, "yVert"=-854.8, "zVert"=30.0, "xNorm"=0.0, "yNorm"=0.0, "zNorm"=-1.0, "BuildIndex"=26}, {"xVert"=-1197.05, "yVert"=-769.2, "zVert"=30.0, "xNorm"=0.0, "yNorm"=0.0, "zNorm"=-1.0, "BuildIndex"=27}, {"xVert"=-1197.05, "yVert"=-769.2, "zVert"=0.0, "xNorm"=0.0, "yNorm"=0.0, "zNorm"=-1.0, "BuildIndex"=27}, {"xVert"=-1197.05, "yVert"=-962.2, "zVert"=0.0, "xNorm"=0.0, "yNorm"=0.0, "zNorm"=-1.0, "BuildIndex"=27}, {"xVert"=-1097.05, "yVert"=-962.2, "zVert"=0.0, "xNorm"=0.0, "yNorm"=0.0, "zNorm"=-1.0, "BuildIndex"=27}, {"xVert"=-1097.05, "yVert"=-1039.2, "zVert"=0.0, "xNorm"=0.0, "yNorm"=0.0, "zNorm"=-1.0, "BuildIndex"=27}, {"xVert"=-1492.05, "yVert"=-1039.2, "zVert"=0.0, "xNorm"=0.0, "yNorm"=0.0, "zNorm"=-1.0, "BuildIndex"=27}, {"xVert"=-1492.05, "yVert"=-769.2, "zVert"=0.0, "xNorm"=0.0, "yNorm"=0.0, "zNorm"=-1.0, "BuildIndex"=27}, {"xVert"=-1197.05, "yVert"=-769.2, "zVert"=0.0, "xNorm"=0.0, "yNorm"=0.0, "zNorm"=-1.0, "BuildIndex"=27}, {"xVert"=-1197.05, "yVert"=-769.2, "zVert"=30.0, "xNorm"=0.0, "yNorm"=0.0, "zNorm"=-1.0, "BuildIndex"=27}, {"xVert"=-268.0, "yVert"=-1099.95, "zVert"=30.0, "xNorm"=0.0, "yNorm"=0.0, "zNorm"=-1.0, "BuildIndex"=28}, {"xVert"=-268.0, "yVert"=-1099.95, "zVert"=0.0, "xNorm"=0.0, "yNorm"=0.0, "zNorm"=-1.0, "BuildIndex"=28}, {"xVert"=-53.0, "yVert"=-1099.95, "zVert"=0.0, "xNorm"=0.0, "yNorm"=0.0, "zNorm"=-1.0, "BuildIndex"=28}, {"xVert"=-53.0, "yVert"=-1489.95, "zVert"=0.0, "xNorm"=0.0, "yNorm"=0.0, "zNorm"=-1.0, "BuildIndex"=28}, {"xVert"=-268.0, "yVert"=-1489.95, "zVert"=0.0, "xNorm"=0.0, "yNorm"=0.0, "zNorm"=-1.0, "BuildIndex"=28}, {"xVert"=-268.0, "yVert"=-1099.95, "zVert"=0.0, "xNorm"=0.0, "yNorm"=0.0, "zNorm"=-1.0, "BuildIndex"=28}, {"xVert"=-268.0, "yVert"=-1099.95, "zVert"=30.0, "xNorm"=0.0, "yNorm"=0.0, "zNorm"=-1.0, "BuildIndex"=28}, {"xVert"=-484.25, "yVert"=-1099.95, "zVert"=30.0, "xNorm"=0.0, "yNorm"=0.0, "zNorm"=-1.0, "BuildIndex"=29}, {"xVert"=-484.25, "yVert"=-1099.95, "zVert"=0.0, "xNorm"=0.0, "yNorm"=0.0, "zNorm"=-1.0, "BuildIndex"=29}, {"xVert"=-284.25, "yVert"=-1099.95, "zVert"=0.0, "xNorm"=0.0, "yNorm"=0.0, "zNorm"=-1.0, "BuildIndex"=29}, {"xVert"=-284.25, "yVert"=-1489.95, "zVert"=0.0, "xNorm"=0.0, "yNorm"=0.0, "zNorm"=-1.0, "BuildIndex"=29}, {"xVert"=-484.25, "yVert"=-1489.95, "zVert"=0.0, "xNorm"=0.0, "yNorm"=0.0, "zNorm"=-1.0, "BuildIndex"=29}, {"xVert"=-484.25, "yVert"=-1099.95, "zVert"=0.0, "xNorm"=0.0, "yNorm"=0.0, "zNorm"=-1.0, "BuildIndex"=29}, {"xVert"=-484.25, "yVert"=-1099.95, "zVert"=30.0, "xNorm"=0.0, "yNorm"=0.0, "zNorm"=-1.0, "BuildIndex"=29}, {"xVert"=-1001.75, "yVert"=-1098.0, "zVert"=30.0, "xNorm"=0.0, "yNorm"=0.0, "zNorm"=-1.0, "BuildIndex"=30}, {"xVert"=-1001.75, "yVert"=-1098.0, "zVert"=0.0, "xNorm"=0.0, "yNorm"=0.0, "zNorm"=-1.0, "BuildIndex"=30}, {"xVert"=-576.75, "yVert"=-1098.0, "zVert"=0.0, "xNorm"=0.0, "yNorm"=0.0, "zNorm"=-1.0, "BuildIndex"=30}, {"xVert"=-576.75, "yVert"=-1478.0, "zVert"=0.0, "xNorm"=0.0, "yNorm"=0.0, "zNorm"=-1.0, "BuildIndex"=30}, {"xVert"=-1001.75, "yVert"=-1478.0, "zVert"=0.0, "xNorm"=0.0, "yNorm"=0.0, "zNorm"=-1.0, "BuildIndex"=30}, {"xVert"=-1001.75, "yVert"=-1098.0, "zVert"=0.0, "xNorm"=0.0, "yNorm"=0.0, "zNorm"=-1.0, "BuildIndex"=30}, {"xVert"=-1001.75, "yVert"=-1098.0, "zVert"=30.0, "xNorm"=0.0, "yNorm"=0.0, "zNorm"=-1.0, "BuildIndex"=30}, {"xVert"=-1488.2, "yVert"=-1098.0, "zVert"=30.0, "xNorm"=0.0, "yNorm"=0.0, "zNorm"=-1.0, "BuildIndex"=31}, {"xVert"=-1488.2, "yVert"=-1098.0, "zVert"=0.0, "xNorm"=0.0, "yNorm"=0.0, "zNorm"=-1.0, "BuildIndex"=31}, {"xVert"=-1098.2, "yVert"=-1098.0, "zVert"=0.0, "xNorm"=0.0, "yNorm"=0.0, "zNorm"=-1.0, "BuildIndex"=31}, {"xVert"=-1098.2, "yVert"=-1468.0, "zVert"=0.0, "xNorm"=0.0, "yNorm"=0.0, "zNorm"=-1.0, "BuildIndex"=31}, {"xVert"=-1488.2, "yVert"=-1468.0, "zVert"=0.0, "xNorm"=0.0, "yNorm"=0.0, "zNorm"=-1.0, "BuildIndex"=31}, {"xVert"=-1488.2, "yVert"=-1098.0, "zVert"=0.0, "xNorm"=0.0, "yNorm"=0.0, "zNorm"=-1.0, "BuildIndex"=31}, {"xVert"=-1488.2, "yVert"=-1098.0, "zVert"=30.0, "xNorm"=0.0, "yNorm"=0.0, "zNorm"=-1.0, "BuildIndex"=31}, {"xVert"=-884.6, "yVert"=-1019.23, "zVert"=30.0, "xNorm"=0.0, "yNorm"=0.0, "zNorm"=-1.0, "BuildIndex"=32}, {"xVert"=-884.6, "yVert"=-1019.23, "zVert"=0.0, "xNorm"=0.0, "yNorm"=0.0, "zNorm"=-1.0, "BuildIndex"=32}, {"xVert"=-997.1, "yVert"=-1019.23, "zVert"=0.0, "xNorm"=0.0, "yNorm"=0.0, "zNorm"=-1.0, "BuildIndex"=32}, {"xVert"=-997.1, "yVert"=-940.73, "zVert"=0.0, "xNorm"=0.0, "yNorm"=0.0, "zNorm"=-1.0, "BuildIndex"=32}, {"xVert"=-884.6, "yVert"=-940.73, "zVert"=0.0, "xNorm"=0.0, "yNorm"=0.0, "zNorm"=-1.0, "BuildIndex"=32}, {"xVert"=-884.6, "yVert"=-1019.23, "zVert"=0.0, "xNorm"=0.0, "yNorm"=0.0, "zNorm"=-1.0, "BuildIndex"=32}, {"xVert"=-884.6, "yVert"=-1019.23, "zVert"=30.0, "xNorm"=0.0, "yNorm"=0.0, "zNorm"=-1.0, "BuildIndex"=32}, {"xVert"=-884.0, "yVert"=-930.0, "zVert"=30.0, "xNorm"=0.0, "yNorm"=0.0, "zNorm"=-1.0, "BuildIndex"=33}, {"xVert"=-884.0, "yVert"=-930.0, "zVert"=0.0, "xNorm"=0.0, "yNorm"=0.0, "zNorm"=-1.0, "BuildIndex"=33}, {"xVert"=-884.0, "yVert"=-755.0, "zVert"=0.0, "xNorm"=0.0, "yNorm"=0.0, "zNorm"=-1.0, "BuildIndex"=33}, {"xVert"=-567.0, "yVert"=-755.0, "zVert"=0.0, "xNorm"=0.0, "yNorm"=0.0, "zNorm"=-1.0, "BuildIndex"=33}, {"xVert"=-567.0, "yVert"=-1019.0, "zVert"=0.0, "xNorm"=0.0, "yNorm"=0.0, "zNorm"=-1.0, "BuildIndex"=33}, {"xVert"=-884.0, "yVert"=-1019.0, "zVert"=0.0, "xNorm"=0.0, "yNorm"=0.0, "zNorm"=-1.0, "BuildIndex"=33}, {"xVert"=-884.0, "yVert"=-930.0, "zVert"=0.0, "xNorm"=0.0, "yNorm"=0.0, "zNorm"=-1.0, "BuildIndex"=33}, {"xVert"=-884.0, "yVert"=-930.0, "zVert"=30.0, "xNorm"=0.0, "yNorm"=0.0, "zNorm"=-1.0, "BuildIndex"=33}, {"xVert"=53.0, "yVert"=-1489.95, "zVert"=30.0, "xNorm"=0.0, "yNorm"=0.0, "zNorm"=-1.0, "BuildIndex"=34}, {"xVert"=53.0, "yVert"=-1489.95, "zVert"=0.0, "xNorm"=0.0, "yNorm"=0.0, "zNorm"=-1.0, "BuildIndex"=34}, {"xVert"=53.0, "yVert"=-1099.95, "zVert"=0.0, "xNorm"=0.0, "yNorm"=0.0, "zNorm"=-1.0, "BuildIndex"=34}, {"xVert"=213.0, "yVert"=-1099.95, "zVert"=0.0, "xNorm"=0.0, "yNorm"=0.0, "zNorm"=-1.0, "BuildIndex"=34}, {"xVert"=213.0, "yVert"=-1489.95, "zVert"=0.0, "xNorm"=0.0, "yNorm"=0.0, "zNorm"=-1.0, "BuildIndex"=34}, {"xVert"=53.0, "yVert"=-1489.95, "zVert"=0.0, "xNorm"=0.0, "yNorm"=0.0, "zNorm"=-1.0, "BuildIndex"=34}, {"xVert"=53.0, "yVert"=-1489.95, "zVert"=30.0, "xNorm"=0.0, "yNorm"=0.0, "zNorm"=-1.0, "BuildIndex"=34}, {"xVert"=235.55, "yVert"=-1489.95, "zVert"=30.0, "xNorm"=0.0, "yNorm"=0.0, "zNorm"=-1.0, "BuildIndex"=35}, {"xVert"=235.55, "yVert"=-1489.95, "zVert"=0.0, "xNorm"=0.0, "yNorm"=0.0, "zNorm"=-1.0, "BuildIndex"=35}, {"xVert"=235.55, "yVert"=-1099.95, "zVert"=0.0, "xNorm"=0.0, "yNorm"=0.0, "zNorm"=-1.0, "BuildIndex"=35}, {"xVert"=360.55, "yVert"=-1099.95, "zVert"=0.0, "xNorm"=0.0, "yNorm"=0.0, "zNorm"=-1.0, "BuildIndex"=35}, {"xVert"=360.55, "yVert"=-1489.95, "zVert"=0.0, "xNorm"=0.0, "yNorm"=0.0, "zNorm"=-1.0, "BuildIndex"=35}, {"xVert"=235.55, "yVert"=-1489.95, "zVert"=0.0, "xNorm"=0.0, "yNorm"=0.0, "zNorm"=-1.0, "BuildIndex"=35}, {"xVert"=235.55, "yVert"=-1489.95, "zVert"=30.0, "xNorm"=0.0, "yNorm"=0.0, "zNorm"=-1.0, "BuildIndex"=35}, {"xVert"=418.25, "yVert"=-1099.95, "zVert"=30.0, "xNorm"=0.0, "yNorm"=0.0, "zNorm"=-1.0, "BuildIndex"=36}, {"xVert"=418.25, "yVert"=-1099.95, "zVert"=0.0, "xNorm"=0.0, "yNorm"=0.0, "zNorm"=-1.0, "BuildIndex"=36}, {"xVert"=718.25, "yVert"=-1099.95, "zVert"=0.0, "xNorm"=0.0, "yNorm"=0.0, "zNorm"=-1.0, "BuildIndex"=36}, {"xVert"=718.25, "yVert"=-1489.95, "zVert"=0.0, "xNorm"=0.0, "yNorm"=0.0, "zNorm"=-1.0, "BuildIndex"=36}, {"xVert"=418.25, "yVert"=-1489.95, "zVert"=0.0, "xNorm"=0.0, "yNorm"=0.0, "zNorm"=-1.0, "BuildIndex"=36}, {"xVert"=418.25, "yVert"=-1099.95, "zVert"=0.0, "xNorm"=0.0, "yNorm"=0.0, "zNorm"=-1.0, "BuildIndex"=36}, {"xVert"=418.25, "yVert"=-1099.95, "zVert"=30.0, "xNorm"=0.0, "yNorm"=0.0, "zNorm"=-1.0, "BuildIndex"=36}, {"xVert"=826.9, "yVert"=-1099.95, "zVert"=30.0, "xNorm"=0.0, "yNorm"=0.0, "zNorm"=-1.0, "BuildIndex"=37}, {"xVert"=826.9, "yVert"=-1099.95, "zVert"=0.0, "xNorm"=0.0, "yNorm"=0.0, "zNorm"=-1.0, "BuildIndex"=37}, {"xVert"=971.9, "yVert"=-1099.95, "zVert"=0.0, "xNorm"=0.0, "yNorm"=0.0, "zNorm"=-1.0, "BuildIndex"=37}, {"xVert"=971.9, "yVert"=-1489.95, "zVert"=0.0, "xNorm"=0.0, "yNorm"=0.0, "zNorm"=-1.0, "BuildIndex"=37}, {"xVert"=826.9, "yVert"=-1489.95, "zVert"=0.0, "xNorm"=0.0, "yNorm"=0.0, "zNorm"=-1.0, "BuildIndex"=37}, {"xVert"=826.9, "yVert"=-1099.95, "zVert"=0.0, "xNorm"=0.0, "yNorm"=0.0, "zNorm"=-1.0, "BuildIndex"=37}, {"xVert"=826.9, "yVert"=-1099.95, "zVert"=30.0, "xNorm"=0.0, "yNorm"=0.0, "zNorm"=-1.0, "BuildIndex"=37}, {"xVert"=1000.0, "yVert"=-1489.95, "zVert"=30.0, "xNorm"=0.0, "yNorm"=0.0, "zNorm"=-1.0, "BuildIndex"=38}, {"xVert"=1000.0, "yVert"=-1489.95, "zVert"=0.0, "xNorm"=0.0, "yNorm"=0.0, "zNorm"=-1.0, "BuildIndex"=38}, {"xVert"=1000.0, "yVert"=-1099.95, "zVert"=0.0, "xNorm"=0.0, "yNorm"=0.0, "zNorm"=-1.0, "BuildIndex"=38}, {"xVert"=1115.0, "yVert"=-1099.95, "zVert"=0.0, "xNorm"=0.0, "yNorm"=0.0, "zNorm"=-1.0, "BuildIndex"=38}, {"xVert"=1130.0, "yVert"=-1489.95, "zVert"=0.0, "xNorm"=0.0, "yNorm"=0.0, "zNorm"=-1.0, "BuildIndex"=38}, {"xVert"=1000.0, "yVert"=-1489.95, "zVert"=0.0, "xNorm"=0.0, "yNorm"=0.0, "zNorm"=-1.0, "BuildIndex"=38}, {"xVert"=1000.0, "yVert"=-1489.95, "zVert"=30.0, "xNorm"=0.0, "yNorm"=0.0, "zNorm"=-1.0, "BuildIndex"=38}, {"xVert"=-38.0, "yVert"=500.0, "zVert"=30.0, "xNorm"=0.0, "yNorm"=0.0, "zNorm"=-1.0, "BuildIndex"=39}, {"xVert"=-38.0, "yVert"=500.0, "zVert"=0.0, "xNorm"=0.0, "yNorm"=0.0, "zNorm"=-1.0, "BuildIndex"=39}, {"xVert"=-38.0, "yVert"=279.0, "zVert"=0.0, "xNorm"=0.0, "yNorm"=0.0, "zNorm"=-1.0, "BuildIndex"=39}, {"xVert"=-490.0, "yVert"=279.0, "zVert"=0.0, "xNorm"=0.0, "yNorm"=0.0, "zNorm"=-1.0, "BuildIndex"=39}, {"xVert"=-490.0, "yVert"=500.0, "zVert"=0.0, "xNorm"=0.0, "yNorm"=0.0, "zNorm"=-1.0, "BuildIndex"=39}, {"xVert"=-38.0, "yVert"=500.0, "zVert"=0.0, "xNorm"=0.0, "yNorm"=0.0, "zNorm"=-1.0, "BuildIndex"=39}, {"xVert"=-38.0, "yVert"=500.0, "zVert"=30.0, "xNorm"=0.0, "yNorm"=0.0, "zNorm"=-1.0, "BuildIndex"=39}, {"xVert"=-476.0, "yVert"=-135.0, "zVert"=30.0, "xNorm"=0.0, "yNorm"=0.0, "zNorm"=-1.0, "BuildIndex"=40}, {"xVert"=-476.0, "yVert"=-135.0, "zVert"=0.0, "xNorm"=0.0, "yNorm"=0.0, "zNorm"=-1.0, "BuildIndex"=40}, {"xVert"=-361.0, "yVert"=-135.0, "zVert"=0.0, "xNorm"=0.0, "yNorm"=0.0, "zNorm"=-1.0, "BuildIndex"=40}, {"xVert"=-361.0, "yVert"=-318.0, "zVert"=0.0, "xNorm"=0.0, "yNorm"=0.0, "zNorm"=-1.0, "BuildIndex"=40}, {"xVert"=-476.0, "yVert"=-318.0, "zVert"=0.0, "xNorm"=0.0, "yNorm"=0.0, "zNorm"=-1.0, "BuildIndex"=40}, {"xVert"=-476.0, "yVert"=-135.0, "zVert"=0.0, "xNorm"=0.0, "yNorm"=0.0, "zNorm"=-1.0, "BuildIndex"=40}, {"xVert"=-476.0, "yVert"=-135.0, "zVert"=30.0, "xNorm"=0.0, "yNorm"=0.0, "zNorm"=-1.0, "BuildIndex"=40}, {"xVert"=-313.0, "yVert"=-135.0, "zVert"=30.0, "xNorm"=0.0, "yNorm"=0.0, "zNorm"=-1.0, "BuildIndex"=41}, {"xVert"=-313.0, "yVert"=-135.0, "zVert"=0.0, "xNorm"=0.0, "yNorm"=0.0, "zNorm"=-1.0, "BuildIndex"=41}, {"xVert"=-58.0, "yVert"=-135.0, "zVert"=0.0, "xNorm"=0.0, "yNorm"=0.0, "zNorm"=-1.0, "BuildIndex"=41}, {"xVert"=-58.0, "yVert"=-308.0, "zVert"=0.0, "xNorm"=0.0, "yNorm"=0.0, "zNorm"=-1.0, "BuildIndex"=41}, {"xVert"=-313.0, "yVert"=-308.0, "zVert"=0.0, "xNorm"=0.0, "yNorm"=0.0, "zNorm"=-1.0, "BuildIndex"=41}, {"xVert"=-313.0, "yVert"=-135.0, "zVert"=0.0, "xNorm"=0.0, "yNorm"=0.0, "zNorm"=-1.0, "BuildIndex"=41}, {"xVert"=-313.0, "yVert"=-135.0, "zVert"=30.0, "xNorm"=0.0, "yNorm"=0.0, "zNorm"=-1.0, "BuildIndex"=41}, {"xVert"=67.0, "yVert"=-130.0, "zVert"=30.0, "xNorm"=0.0, "yNorm"=0.0, "zNorm"=-1.0, "BuildIndex"=42}, {"xVert"=67.0, "yVert"=-130.0, "zVert"=0.0, "xNorm"=0.0, "yNorm"=0.0, "zNorm"=-1.0, "BuildIndex"=42}, {"xVert"=721.0, "yVert"=-130.0, "zVert"=0.0, "xNorm"=0.0, "yNorm"=0.0, "zNorm"=-1.0, "BuildIndex"=42}, {"xVert"=721.0, "yVert"=-318.0, "zVert"=0.0, "xNorm"=0.0, "yNorm"=0.0, "zNorm"=-1.0, "BuildIndex"=42}, {"xVert"=67.0, "yVert"=-318.0, "zVert"=0.0, "xNorm"=0.0, "yNorm"=0.0, "zNorm"=-1.0, "BuildIndex"=42}, {"xVert"=67.0, "yVert"=-130.0, "zVert"=0.0, "xNorm"=0.0, "yNorm"=0.0, "zNorm"=-1.0, "BuildIndex"=42}, {"xVert"=67.0, "yVert"=-130.0, "zVert"=30.0, "xNorm"=0.0, "yNorm"=0.0, "zNorm"=-1.0, "BuildIndex"=42}, {"xVert"=-481.0, "yVert"=-356.0, "zVert"=30.0, "xNorm"=0.0, "yNorm"=0.0, "zNorm"=-1.0, "BuildIndex"=43}, {"xVert"=-481.0, "yVert"=-356.0, "zVert"=0.0, "xNorm"=0.0, "yNorm"=0.0, "zNorm"=-1.0, "BuildIndex"=43}, {"xVert"=-293.0, "yVert"=-356.0, "zVert"=0.0, "xNorm"=0.0, "yNorm"=0.0, "zNorm"=-1.0, "BuildIndex"=43}, {"xVert"=-293.0, "yVert"=-683.0, "zVert"=0.0, "xNorm"=0.0, "yNorm"=0.0, "zNorm"=-1.0, "BuildIndex"=43}, {"xVert"=-481.0, "yVert"=-683.0, "zVert"=0.0, "xNorm"=0.0, "yNorm"=0.0, "zNorm"=-1.0, "BuildIndex"=43}, {"xVert"=-481.0, "yVert"=-356.0, "zVert"=0.0, "xNorm"=0.0, "yNorm"=0.0, "zNorm"=-1.0, "BuildIndex"=43}, {"xVert"=-481.0, "yVert"=-356.0, "zVert"=30.0, "xNorm"=0.0, "yNorm"=0.0, "zNorm"=-1.0, "BuildIndex"=43}, {"xVert"=-260.0, "yVert"=-356.0, "zVert"=30.0, "xNorm"=0.0, "yNorm"=0.0, "zNorm"=-1.0, "BuildIndex"=44}, {"xVert"=-260.0, "yVert"=-356.0, "zVert"=0.0, "xNorm"=0.0, "yNorm"=0.0, "zNorm"=-1.0, "BuildIndex"=44}, {"xVert"=-48.0, "yVert"=-356.0, "zVert"=0.0, "xNorm"=0.0, "yNorm"=0.0, "zNorm"=-1.0, "BuildIndex"=44}, {"xVert"=-48.0, "yVert"=-673.0, "zVert"=0.0, "xNorm"=0.0, "yNorm"=0.0, "zNorm"=-1.0, "BuildIndex"=44}, {"xVert"=-260.0, "yVert"=-673.0, "zVert"=0.0, "xNorm"=0.0, "yNorm"=0.0, "zNorm"=-1.0, "BuildIndex"=44}, {"xVert"=-260.0, "yVert"=-356.0, "zVert"=0.0, "xNorm"=0.0, "yNorm"=0.0, "zNorm"=-1.0, "BuildIndex"=44}, {"xVert"=-260.0, "yVert"=-356.0, "zVert"=30.0, "xNorm"=0.0, "yNorm"=0.0, "zNorm"=-1.0, "BuildIndex"=44}, {"xVert"=558.0, "yVert"=-406.0, "zVert"=30.0, "xNorm"=0.0, "yNorm"=0.0, "zNorm"=-1.0, "BuildIndex"=45}, {"xVert"=558.0, "yVert"=-406.0, "zVert"=0.0, "xNorm"=0.0, "yNorm"=0.0, "zNorm"=-1.0, "BuildIndex"=45}, {"xVert"=712.0, "yVert"=-404.0, "zVert"=0.0, "xNorm"=0.0, "yNorm"=0.0, "zNorm"=-1.0, "BuildIndex"=45}, {"xVert"=712.0, "yVert"=-668.0, "zVert"=0.0, "xNorm"=0.0, "yNorm"=0.0, "zNorm"=-1.0, "BuildIndex"=45}, {"xVert"=58.0, "yVert"=-668.0, "zVert"=0.0, "xNorm"=0.0, "yNorm"=0.0, "zNorm"=-1.0, "BuildIndex"=45}, {"xVert"=58.0, "yVert"=-404.0, "zVert"=0.0, "xNorm"=0.0, "yNorm"=0.0, "zNorm"=-1.0, "BuildIndex"=45}, {"xVert"=154.0, "yVert"=-404.0, "zVert"=0.0, "xNorm"=0.0, "yNorm"=0.0, "zNorm"=-1.0, "BuildIndex"=45}, {"xVert"=154.0, "yVert"=-577.0, "zVert"=0.0, "xNorm"=0.0, "yNorm"=0.0, "zNorm"=-1.0, "BuildIndex"=45}, {"xVert"=558.0, "yVert"=-577.0, "zVert"=0.0, "xNorm"=0.0, "yNorm"=0.0, "zNorm"=-1.0, "BuildIndex"=45}, {"xVert"=558.0, "yVert"=-406.0, "zVert"=0.0, "xNorm"=0.0, "yNorm"=0.0, "zNorm"=-1.0, "BuildIndex"=45}, {"xVert"=558.0, "yVert"=-406.0, "zVert"=30.0, "xNorm"=0.0, "yNorm"=0.0, "zNorm"=-1.0, "BuildIndex"=45}, {"xVert"=173.0, "yVert"=-404.0, "zVert"=30.0, "xNorm"=0.0, "yNorm"=0.0, "zNorm"=-1.0, "BuildIndex"=46}, {"xVert"=173.0, "yVert"=-404.0, "zVert"=0.0, "xNorm"=0.0, "yNorm"=0.0, "zNorm"=-1.0, "BuildIndex"=46}, {"xVert"=534.0, "yVert"=-404.0, "zVert"=0.0, "xNorm"=0.0, "yNorm"=0.0, "zNorm"=-1.0, "BuildIndex"=46}, {"xVert"=534.0, "yVert"=-524.0, "zVert"=0.0, "xNorm"=0.0, "yNorm"=0.0, "zNorm"=-1.0, "BuildIndex"=46}, {"xVert"=173.0, "yVert"=-524.0, "zVert"=0.0, "xNorm"=0.0, "yNorm"=0.0, "zNorm"=-1.0, "BuildIndex"=46}, {"xVert"=173.0, "yVert"=-404.0, "zVert"=0.0, "xNorm"=0.0, "yNorm"=0.0, "zNorm"=-1.0, "BuildIndex"=46}, {"xVert"=173.0, "yVert"=-404.0, "zVert"=30.0, "xNorm"=0.0, "yNorm"=0.0, "zNorm"=-1.0, "BuildIndex"=46}, {"xVert"=-702.0, "yVert"=-115.0, "zVert"=30.0, "xNorm"=0.0, "yNorm"=0.0, "zNorm"=-1.0, "BuildIndex"=47}, {"xVert"=-702.0, "yVert"=-115.0, "zVert"=0.0, "xNorm"=0.0, "yNorm"=0.0, "zNorm"=-1.0, "BuildIndex"=47}, {"xVert"=-567.0, "yVert"=-115.0, "zVert"=0.0, "xNorm"=0.0, "yNorm"=0.0, "zNorm"=-1.0, "BuildIndex"=47}, {"xVert"=-567.0, "yVert"=-673.0, "zVert"=0.0, "xNorm"=0.0, "yNorm"=0.0, "zNorm"=-1.0, "BuildIndex"=47}, {"xVert"=-702.0, "yVert"=-673.0, "zVert"=0.0, "xNorm"=0.0, "yNorm"=0.0, "zNorm"=-1.0, "BuildIndex"=47}, {"xVert"=-702.0, "yVert"=-115.0, "zVert"=0.0, "xNorm"=0.0, "yNorm"=0.0, "zNorm"=-1.0, "BuildIndex"=47}, {"xVert"=-702.0, "yVert"=-115.0, "zVert"=30.0, "xNorm"=0.0, "yNorm"=0.0, "zNorm"=-1.0, "BuildIndex"=47}, {"xVert"=-779.0, "yVert"=495.0, "zVert"=30.0, "xNorm"=0.0, "yNorm"=0.0, "zNorm"=-1.0, "BuildIndex"=48}, {"xVert"=-779.0, "yVert"=495.0, "zVert"=0.0, "xNorm"=0.0, "yNorm"=0.0, "zNorm"=-1.0, "BuildIndex"=48}, {"xVert"=-572.0, "yVert"=495.0, "zVert"=0.0, "xNorm"=0.0, "yNorm"=0.0, "zNorm"=-1.0, "BuildIndex"=48}, {"xVert"=-572.0, "yVert"=82.0, "zVert"=0.0, "xNorm"=0.0, "yNorm"=0.0, "zNorm"=-1.0, "BuildIndex"=48}, {"xVert"=-779.0, "yVert"=82.0, "zVert"=0.0, "xNorm"=0.0, "yNorm"=0.0, "zNorm"=-1.0, "BuildIndex"=48}, {"xVert"=-779.0, "yVert"=495.0, "zVert"=0.0, "xNorm"=0.0, "yNorm"=0.0, "zNorm"=-1.0, "BuildIndex"=48}, {"xVert"=-779.0, "yVert"=495.0, "zVert"=30.0, "xNorm"=0.0, "yNorm"=0.0, "zNorm"=-1.0, "BuildIndex"=48}, {"xVert"=-899.0, "yVert"=-106.0, "zVert"=30.0, "xNorm"=0.0, "yNorm"=0.0, "zNorm"=-1.0, "BuildIndex"=49}, {"xVert"=-899.0, "yVert"=-106.0, "zVert"=0.0, "xNorm"=0.0, "yNorm"=0.0, "zNorm"=-1.0, "BuildIndex"=49}, {"xVert"=-760.0, "yVert"=-106.0, "zVert"=0.0, "xNorm"=0.0, "yNorm"=0.0, "zNorm"=-1.0, "BuildIndex"=49}, {"xVert"=-760.0, "yVert"=-289.0, "zVert"=0.0, "xNorm"=0.0, "yNorm"=0.0, "zNorm"=-1.0, "BuildIndex"=49}, {"xVert"=-899.0, "yVert"=-289.0, "zVert"=0.0, "xNorm"=0.0, "yNorm"=0.0, "zNorm"=-1.0, "BuildIndex"=49}, {"xVert"=-899.0, "yVert"=-106.0, "zVert"=0.0, "xNorm"=0.0, "yNorm"=0.0, "zNorm"=-1.0, "BuildIndex"=49}, {"xVert"=-899.0, "yVert"=-106.0, "zVert"=30.0, "xNorm"=0.0, "yNorm"=0.0, "zNorm"=-1.0, "BuildIndex"=49}, {"xVert"=-500.0, "yVert"=635.0, "zVert"=30.0, "xNorm"=0.0, "yNorm"=0.0, "zNorm"=-1.0, "BuildIndex"=50}, {"xVert"=-500.0, "yVert"=635.0, "zVert"=0.0, "xNorm"=0.0, "yNorm"=0.0, "zNorm"=-1.0, "BuildIndex"=50}, {"xVert"=-500.0, "yVert"=740.0, "zVert"=0.0, "xNorm"=0.0, "yNorm"=0.0, "zNorm"=-1.0, "BuildIndex"=50}, {"xVert"=-433.0, "yVert"=798.0, "zVert"=0.0, "xNorm"=0.0, "yNorm"=0.0, "zNorm"=-1.0, "BuildIndex"=50}, {"xVert"=-106.0, "yVert"=798.0, "zVert"=0.0, "xNorm"=0.0, "yNorm"=0.0, "zNorm"=-1.0, "BuildIndex"=50}, {"xVert"=-38.0, "yVert"=740.0, "zVert"=0.0, "xNorm"=0.0, "yNorm"=0.0, "zNorm"=-1.0, "BuildIndex"=50}, {"xVert"=-38.0, "yVert"=635.0, "zVert"=0.0, "xNorm"=0.0, "yNorm"=0.0, "zNorm"=-1.0, "BuildIndex"=50}, {"xVert"=-106.0, "yVert"=587.0, "zVert"=0.0, "xNorm"=0.0, "yNorm"=0.0, "zNorm"=-1.0, "BuildIndex"=50}, {"xVert"=-433.0, "yVert"=587.0, "zVert"=0.0, "xNorm"=0.0, "yNorm"=0.0, "zNorm"=-1.0, "BuildIndex"=50}, {"xVert"=-500.0, "yVert"=635.0, "zVert"=0.0, "xNorm"=0.0, "yNorm"=0.0, "zNorm"=-1.0, "BuildIndex"=50}, {"xVert"=-500.0, "yVert"=635.0, "zVert"=30.0, "xNorm"=0.0, "yNorm"=0.0, "zNorm"=-1.0, "BuildIndex"=50}, {"xVert"=-48.0, "yVert"=250.0, "zVert"=30.0, "xNorm"=0.0, "yNorm"=0.0, "zNorm"=-1.0, "BuildIndex"=51}, {"xVert"=-48.0, "yVert"=250.0, "zVert"=0.0, "xNorm"=0.0, "yNorm"=0.0, "zNorm"=-1.0, "BuildIndex"=51}, {"xVert"=-48.0, "yVert"=87.0, "zVert"=0.0, "xNorm"=0.0, "yNorm"=0.0, "zNorm"=-1.0, "BuildIndex"=51}, {"xVert"=-490.0, "yVert"=87.0, "zVert"=0.0, "xNorm"=0.0, "yNorm"=0.0, "zNorm"=-1.0, "BuildIndex"=51}, {"xVert"=-490.0, "yVert"=250.0, "zVert"=0.0, "xNorm"=0.0, "yNorm"=0.0, "zNorm"=-1.0, "BuildIndex"=51}, {"xVert"=-48.0, "yVert"=250.0, "zVert"=0.0, "xNorm"=0.0, "yNorm"=0.0, "zNorm"=-1.0, "BuildIndex"=51}, {"xVert"=-48.0, "yVert"=250.0, "zVert"=30.0, "xNorm"=0.0, "yNorm"=0.0, "zNorm"=-1.0, "BuildIndex"=51}] {"zNorm" format="%.2f"; "yNorm" format="%.2f"; "xNorm" format="%.2f"; "zVert" format="%^#_6g"; "yVert" format="%^#_6g"; "xVert" format="%^#_6g"}) -> ()   [LabVIEW 2010]
uses:
  Route mapping/Exclude_cluster.ctl
  Route mapping/Box_size.ctl
  Route mapping/Exclusion_type.ctl
  Traverse_cluster.ctl
  Spacing.ctl
  Controls/Multi_run_mode.ctl
  Controls/Tunnel_Coordinates.ctl
panel:
  out "Row Number":i32=235
  in  "Space file":path=path "/xphayden/Documents/EnFlo_Tunnel/Westlakes_08/Repeat_THORP/Calder1.xls"
  in  "Output Traverse space file":bool
  out "Exclude":T1[](array[typedef])=[{"Sizes"=[{"Max"=337.0, "Min"=58.0}, {"Max"=500.0, "Min"=115.0}, {"Max"=155.0, "Min"=0.0}], "Name"="Block 1", "Exclude Type"=enum."Exclude completely"}, {"Sizes"=[{"Max"=712.0, "Min"=438.0}, {"Max"=490.0, "Min"=91.0}, {"Max"=150.0, "Min"=0.0}], "Name"="Block 2", "Exclude Type"=enum."Exclude completely"}, {"Sizes"=[{"Max"=-764.0, "Min"=-894.0}, {"Max"=-308.0, "Min"=-673.0}, {"Max"=73.0, "Min"=0.0}], "Name"="Block 3", "Exclude Type"=enum."Exclude completely"}, {"Sizes"=[{"Max"=347.0, "Min"=53.0}, {"Max"=1250.0, "Min"=587.0}, {"Max"=108.0, "Min"=0.0}], "Name"="Block 4", "Exclude Type"=enum."Exclude completely"}, {"Sizes"=[{"Max"=510.0, "Min"=442.0}, {"Max"=1250.0, "Min"=596.0}, {"Max"=102.0, "Min"=0.0}], "Name"="Block 5", "Exclude Type"=enum."Exclude completely"}, {"Sizes"=[{"Max"=711.0, "Min"=567.0}, {"Max"=1250.0, "Min"=596.0}, {"Max"=137.0, "Min"=0.0}], "Name"="Block 6", "Exclude Type"=enum."Exclude completely"}, {"Sizes"=[{"Max"=-43.0, "Min"=-485.0}, {"Max"=1043.0, "Min"=889.0}, {"Max"=80.0, "Min"=0.0}], "Name"="Block 7", "Exclude Type"=enum."Exclude completely"}, {"Sizes"=[{"Max"=1086.0, "Min"=822.0}, {"Max"=-130.0, "Min"=-342.0}, {"Max"=100.0, "Min"=0.0}], "Name"="Block 8", "Exclude Type"=enum."Exclude completely"}, {"Sizes"=[{"Max"=707.0, "Min"=433.0}, {"Max"=-750.0, "Min"=-1019.0}, {"Max"=104.0, "Min"=0.0}], "Name"="Block 9", "Exclude Type"=enum."Exclude completely"}, {"Sizes"=[{"Max"=356.0, "Min"=58.0}, {"Max"=-755.0, "Min"=-1019.0}, {"Max"=88.0, "Min"=0.0}], "Name"="Block 10", "Exclude Type"=enum."Exclude completely"}, {"Sizes"=[{"Max"=-48.0, "Min"=-260.0}, {"Max"=-755.0, "Min"=-1019.0}, {"Max"=70.0, "Min"=0.0}], "Name"="Block 11", "Exclude Type"=enum."Exclude completely"}, {"Sizes"=[{"Max"=-279.0, "Min"=-481.0}, {"Max"=-755.0, "Min"=-1019.0}, {"Max"=72.0, "Min"=0.0}], "Name"="Block 12", "Exclude Type"=enum."Exclude completely"}, {"Sizes"=[{"Max"=-966.0, "Min"=-1139.0}, {"Max"=-106.0, "Min"=-683.0}, {"Max"=93.0, "Min"=0.0}], "Name"="Block 13", "Exclude Type"=enum."Exclude completely"}, {"Sizes"=[{"Max"=-885.0, "Min"=-1250.0}, {"Max"=490.0, "Min"=120.0}, {"Max"=168.0, "Min"=0.0}], "Name"="Block 14", "Exclude Type"=enum."Exclude completely"}, {"Sizes"=[{"Max"=-577.0, "Min"=-731.0}, {"Max"=1481.0, "Min"=582.0}, {"Max"=85.0, "Min"=0.0}], "Name"="Block 15", "Exclude Type"=enum."Exclude completely"}, {"Sizes"=[{"Max"=1106.0, "Min"=832.0}, {"Max"=-404.0, "Min"=-1019.0}, {"Max"=75.0, "Min"=0.0}], "Name"="Block 16", "Exclude Type"=enum."Exclude completely"}, {"Sizes"=[{"Max"=1452.0, "Min"=827.0}, {"Max"=1058.0, "Min"=130.0}, {"Max"=159.0, "Min"=0.0}], "Name"="Block 17", "Exclude Type"=enum."Exclude completely"}, {"Sizes"=[{"Max"=-774.0, "Min"=-1337.0}, {"Max"=1635.0, "Min"=663.0}, {"Max"=78.0, "Min"=0.0}], "Name"="Block 18", "Exclude Type"=enum."Exclude completely"}, {"Sizes"=[{"Max"=1404.0, "Min"=1183.0}, {"Max"=-125.0, "Min"=-1019.0}, {"Max"=105.0, "Min"=0.0}], "Name"="Block 19", "Exclude Type"=enum."Exclude completely"}, {"Sizes"=[{"Max"=1885.0, "Min"=1308.0}, {"Max"=-115.0, "Min"=-221.0}, {"Max"=120.0, "Min"=0.0}], "Name"="Block 20", "Exclude Type"=enum."Exclude completely"}, {"Sizes"=[{"Max"=1461.0, "Min"=1389.0}, {"Max"=-274.0, "Min"=-510.0}, {"Max"=100.0, "Min"=0.0}], "Name"="Block 21", "Exclude Type"=enum."Exclude completely"}, {"Sizes"=[{"Max"=1625.0, "Min"=1529.0}, {"Max"=-438.0, "Min"=-520.0}, {"Max"=320.0, "Min"=0.0}], "Name"="Block 22", "Exclude Type"=enum."Exclude completely"}, {"Sizes"=[{"Max"=1625.0, "Min"=1529.0}, {"Max"=-543.0, "Min"=-673.0}, {"Max"=320.0, "Min"=0.0}], "Name"="Block 23", "Exclude Type"=enum."Exclude completely"}, {"Sizes"=[{"Max"=1803.0, "Min"=1558.0}, {"Max"=-255.0, "Min"=-423.0}, {"Max"=75.0, "Min"=0.0}], "Name"="Block 24", "Exclude Type"=enum."Exclude completely"}, {"Sizes"=[{"Max"=2375.0, "Min"=1548.1}, {"Max"=307.69, "Min"=86.54}, {"Max"=95.0, "Min"=0.0}], "Name"="Block 25", "Exclude Type"=enum."Exclude completely"}, {"Sizes"=[{"Max"=-949.55, "Min"=-1139.55}, {"Max"=-754.8, "Min"=-864.8}, {"Max"=67.5, "Min"=0.0}], "Name"="Block 26", "Exclude Type"=enum."Exclude completely"}, {"Sizes"=[{"Max"=-1097.05, "Min"=-1492.05}, {"Max"=-769.2, "Min"=-1039.2}, {"Max"=70.0, "Min"=0.0}], "Name"="Block 27", "Exclude Type"=enum."Exclude completely"}, {"Sizes"=[{"Max"=-53.0, "Min"=-268.0}, {"Max"=-1099.95, "Min"=-1489.95}, {"Max"=90.0, "Min"=0.0}], "Name"="Block 28", "Exclude Type"=enum."Exclude completely"}, {"Sizes"=[{"Max"=-284.25, "Min"=-484.25}, {"Max"=-1099.95, "Min"=-1489.95}, {"Max"=87.5, "Min"=0.0}], "Name"="Block 29", "Exclude Type"=enum."Exclude completely"}, {"Sizes"=[{"Max"=-576.75, "Min"=-1001.75}, {"Max"=-1098.0, "Min"=-1478.0}, {"Max"=90.0, "Min"=0.0}], "Name"="Block 30", "Exclude Type"=enum."Exclude completely"}, {"Sizes"=[{"Max"=-1098.2, "Min"=-1488.2}, {"Max"=-1098.0, "Min"=-1468.0}, {"Max"=100.0, "Min"=0.0}], "Name"="Block 31", "Exclude Type"=enum."Exclude completely"}, {"Sizes"=[{"Max"=-884.6, "Min"=-997.1}, {"Max"=-940.73, "Min"=-1019.23}, {"Max"=70.0, "Min"=0.0}], "Name"="Block 32", "Exclude Type"=enum."Exclude completely"}, {"Sizes"=[{"Max"=-567.0, "Min"=-884.0}, {"Max"=-755.0, "Min"=-1019.0}, {"Max"=70.0, "Min"=0.0}], "Name"="Block 33", "Exclude Type"=enum."Exclude completely"}, {"Sizes"=[{"Max"=213.0, "Min"=53.0}, {"Max"=-1099.95, "Min"=-1489.95}, {"Max"=77.5, "Min"=0.0}], "Name"="Block 34", "Exclude Type"=enum."Exclude completely"}, {"Sizes"=[{"Max"=360.55, "Min"=235.55}, {"Max"=-1099.95, "Min"=-1489.95}, {"Max"=85.0, "Min"=0.0}], "Name"="Block 35", "Exclude Type"=enum."Exclude completely"}, {"Sizes"=[{"Max"=718.25, "Min"=418.25}, {"Max"=-1099.95, "Min"=-1489.95}, {"Max"=82.5, "Min"=0.0}], "Name"="Block 36", "Exclude Type"=enum."Exclude completely"}, {"Sizes"=[{"Max"=971.9, "Min"=826.9}, {"Max"=-1099.95, "Min"=-1489.95}, {"Max"=100.0, "Min"=0.0}], "Name"="Block 37", "Exclude Type"=enum."Exclude completely"}, {"Sizes"=[{"Max"=1130.0, "Min"=1000.0}, {"Max"=-1099.95, "Min"=-1489.95}, {"Max"=70.0, "Min"=0.0}], "Name"="Block 38", "Exclude Type"=enum."Exclude completely"}, {"Sizes"=[{"Max"=-38.0, "Min"=-490.0}, {"Max"=500.0, "Min"=279.0}, {"Max"=88.0, "Min"=0.0}], "Name"="Block 39", "Exclude Type"=enum."Exclude completely"}, {"Sizes"=[{"Max"=-361.0, "Min"=-476.0}, {"Max"=-135.0, "Min"=-318.0}, {"Max"=75.0, "Min"=0.0}], "Name"="Block 40", "Exclude Type"=enum."Exclude completely"}, {"Sizes"=[{"Max"=-58.0, "Min"=-313.0}, {"Max"=-135.0, "Min"=-308.0}, {"Max"=245.0, "Min"=0.0}], "Name"="Block 41", "Exclude Type"=enum."Exclude completely"}, {"Sizes"=[{"Max"=721.0, "Min"=67.0}, {"Max"=-130.0, "Min"=-318.0}, {"Max"=115.0, "Min"=0.0}], "Name"="Block 42", "Exclude Type"=enum."Exclude completely"}, {"Sizes"=[{"Max"=-293.0, "Min"=-481.0}, {"Max"=-356.0, "Min"=-683.0}, {"Max"=68.0, "Min"=0.0}], "Name"="Block 43", "Exclude Type"=enum."Exclude completely"}, {"Sizes"=[{"Max"=-48.0, "Min"=-260.0}, {"Max"=-356.0, "Min"=-673.0}, {"Max"=90.0, "Min"=0.0}], "Name"="Block 44", "Exclude Type"=enum."Exclude completely"}, {"Sizes"=[{"Max"=712.0, "Min"=58.0}, {"Max"=-404.0, "Min"=-668.0}, {"Max"=84.0, "Min"=0.0}], "Name"="Block 45", "Exclude Type"=enum."Exclude completely"}, {"Sizes"=[{"Max"=534.0, "Min"=173.0}, {"Max"=-404.0, "Min"=-524.0}, {"Max"=120.0, "Min"=0.0}], "Name"="Block 46", "Exclude Type"=enum."Exclude completely"}, {"Sizes"=[{"Max"=-567.0, "Min"=-702.0}, {"Max"=-115.0, "Min"=-673.0}, {"Max"=120.0, "Min"=0.0}], "Name"="Block 47", "Exclude Type"=enum."Exclude completely"}, {"Sizes"=[{"Max"=-572.0, "Min"=-779.0}, {"Max"=495.0, "Min"=82.0}, {"Max"=128.0, "Min"=0.0}], "Name"="Block 48", "Exclude Type"=enum."Exclude completely"}, {"Sizes"=[{"Max"=-760.0, "Min"=-899.0}, {"Max"=-106.0, "Min"=-289.0}, {"Max"=125.0, "Min"=0.0}], "Name"="Block 49", "Exclude Type"=enum."Exclude completely"}, {"Sizes"=[{"Max"=-38.0, "Min"=-500.0}, {"Max"=798.0, "Min"=587.0}, {"Max"=0.0, "Min"=0.0}], "Name"="Block 50", "Exclude Type"=enum."Exclude completely"}, {"Sizes"=[{"Max"=-48.0, "Min"=-490.0}, {"Max"=250.0, "Min"=87.0}, {"Max"=265.0, "Min"=0.0}], "Name"="Block 51", "Exclude Type"=enum."Exclude completely"}] {"Sizes"."Min" format="%#.1f"; "Sizes"."Max" format="%#.1f"}
  in  "Trav Space":T4={"X min"=-2000.0, "Xmax"=2500.0, "Ymin"=-850.0, "Y max"=850.0} {"Y max" step=100.0; "Ymin" step=100.0; "Xmax" step=100.0; "X min" step=100.0}
  in  "Coordinate rotation (deg)":dbl=-51.4 format="%.2f"
  in  "millisecond multiple":u32=50
  out "Output File":picture
  out "Raw points":i32=393
  out "points output":i32=390
  in  "Redraw?":bool
  in  "Output Setup file":bool
  in  "Setup filename":path=path "/iMac-Duo-9-HD/Users/paulhayden/Desktop/dapple_floorplan_test.xls"
  out "Plot?":bool
  out "Accept array":u32[](array[numeric])=[1, 2, 3, 4, 5, 6, 7, 8, 9, 10, 11, 12, 13, 14, 15, 16, 17, 18, 19, 20, 21, 22, 23, 24, 25, 26, 27, 28, 29, 30, 31, 32, 33, 34, 35, 36, 37, 38, 39, 40, 41, 42, 43, 44, 45, 46, 47, 48, 49, 50, 51]
  in  "Output rectangle":T4={"X min"=-3000.0, "Xmax"=3000.0, "Ymin"=-3000.0, "Y max"=3000.0} {"Y max" step=100.0; "Ymin" step=100.0; "Xmax" step=100.0; "X min" step=100.0}
  in  "Turntable Diameter (mm)":dbl=3500.0
  in  "stop":bool
  out "Picture":picture
  out "RowNum":i32=394
  out "NumLines":i32=393
  in  "ScaleFactor":dbl=12.0
  in  "Y Centre(mm)":dbl step=100.0
  in  "X Centre(mm)":dbl step=100.0
  # "Horizontal X Axis  positive to the right"
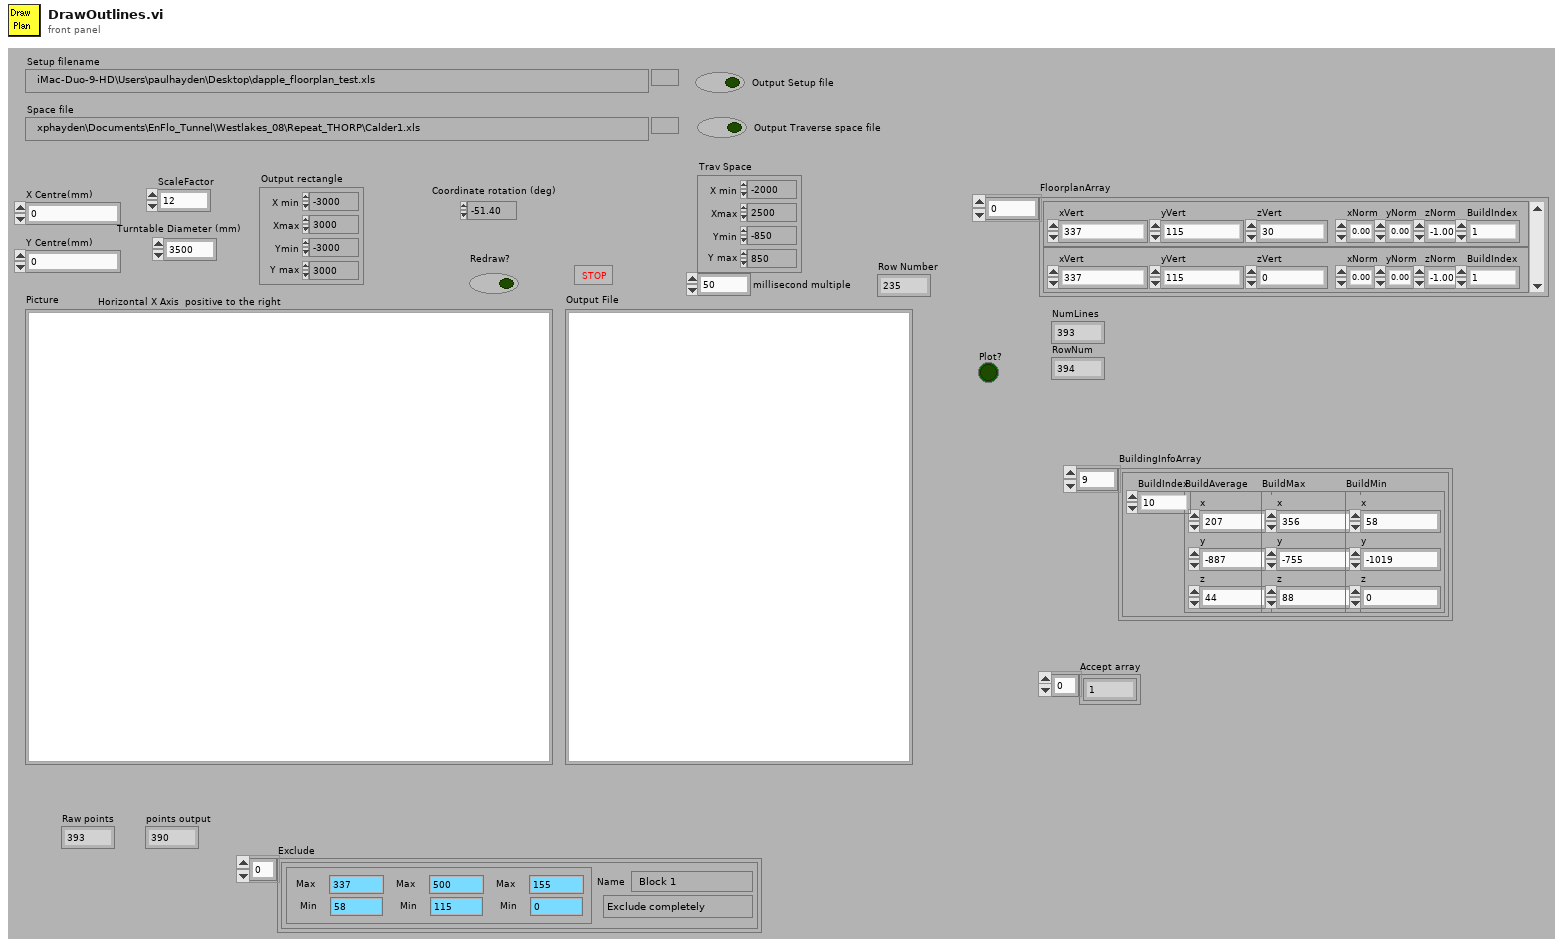
[diagram p1: front panel]
types:
  T1 = typedef "Exclude_cluster.ctl" = cluster{"Sizes":T2, "Name":string, "Exclude Type":T3}
  T2 = typedef "Box_size.ctl" = cluster{"Max":dbl, "Min":dbl}[]
  T3 = typedef "Exclusion_type.ctl" = enum16{"Exclude completely", "Allow only vertical moves"}
  T4 = cluster{"X min":dbl, "Xmax":dbl, "Ymin":dbl, "Y max":dbl}
  T5 = cluster{"BuildAverage":cluster{"x":dbl, "y":dbl, "z":dbl}, "BuildIndex":u32, "BuildMax":cluster{"x":dbl, "y":dbl, "z":dbl}, "BuildMin":cluster{"x":dbl, "y":dbl, "z":dbl}}[]
  T6 = cluster{"xVert":dbl, "yVert":dbl, "zVert":dbl, "xNorm":dbl, "yNorm":dbl, "zNorm":dbl, "BuildIndex":u32}[]
  T7 = typedef "LVBoundsTypeDef.ctl" = cluster{"Width":u32, "Height":u32}
  T8 = cluster{"Width":u16, "Style":enum32{"Solid", "Dash", "Dot", "DashDot", "DashDotDot"}}
  T9 = cluster{"left":i16, "top":i16, "right":i16, "bottom":i16}
  T10 = enum16{"Load setup from excel file", "Save setup to excel file"}
  T11 = enum16{"To Traverse Coordinates", "To User Coordinates"}
  T12 = typedef "Traverse_cluster.ctl" = cluster{"Start X":dbl, "Start Y":dbl, "Start Z":dbl, "End X":dbl, "End Y":dbl, "End Z":dbl, "No. of pts.":i32, "Spacing":T13, "Filename":path, "Tunnel Speed":dbl, "Averaging time (min)":dbl, "Extra Commands":string, "Specific Arguments":string, "Emission Rate (l/min)":dbl, "Trace Gas Concentration (%)":dbl, "Density Ratio":string, "Comments":string, "Row No":i32, "Row Type Selector":T14, "Completion time":string, "Row Duration (mins)":dbl, "No. of Valid pts.":i32, "Meas Setup File":string}
  T13 = typedef "Spacing.ctl" = enum16{"Linear", "Log", "Gauss", "Specified", "N/A"}
  T14 = typedef "Multi_run_mode.ctl" = enum16{"Move Traverse Only", "Set Tunnel Speed Only", "Set Source Only", "Set Measurement Conditions", "Single Measurement", "Vertical Profile", "Lateral Profile", "Longitudinal Profile", "Explore Volume", "Multi-Axis Profile", "Auto Calibrate", "Meas Fast FID Bkgnd", "Check Beam Power", "Scanning Valve Measurement", "Run VI Named:", "Set ADAM Ch", "Wait (minutes)", "Send Message", "Synchronize With:", "Fall Back to this Row", "Turn Off Row Repeating", "Blank Row"}
  T15 = typedef "Tunnel_Coordinates.ctl" = enum16{"Work in Tunnel Coordinates", "Work in Model Coordinates"}
  T16 = cluster{"xVert":dbl, "yVert":dbl, "zVert":dbl, "xNorm":dbl, "yNorm":dbl, "zNorm":dbl, "BuildIndex":u32}
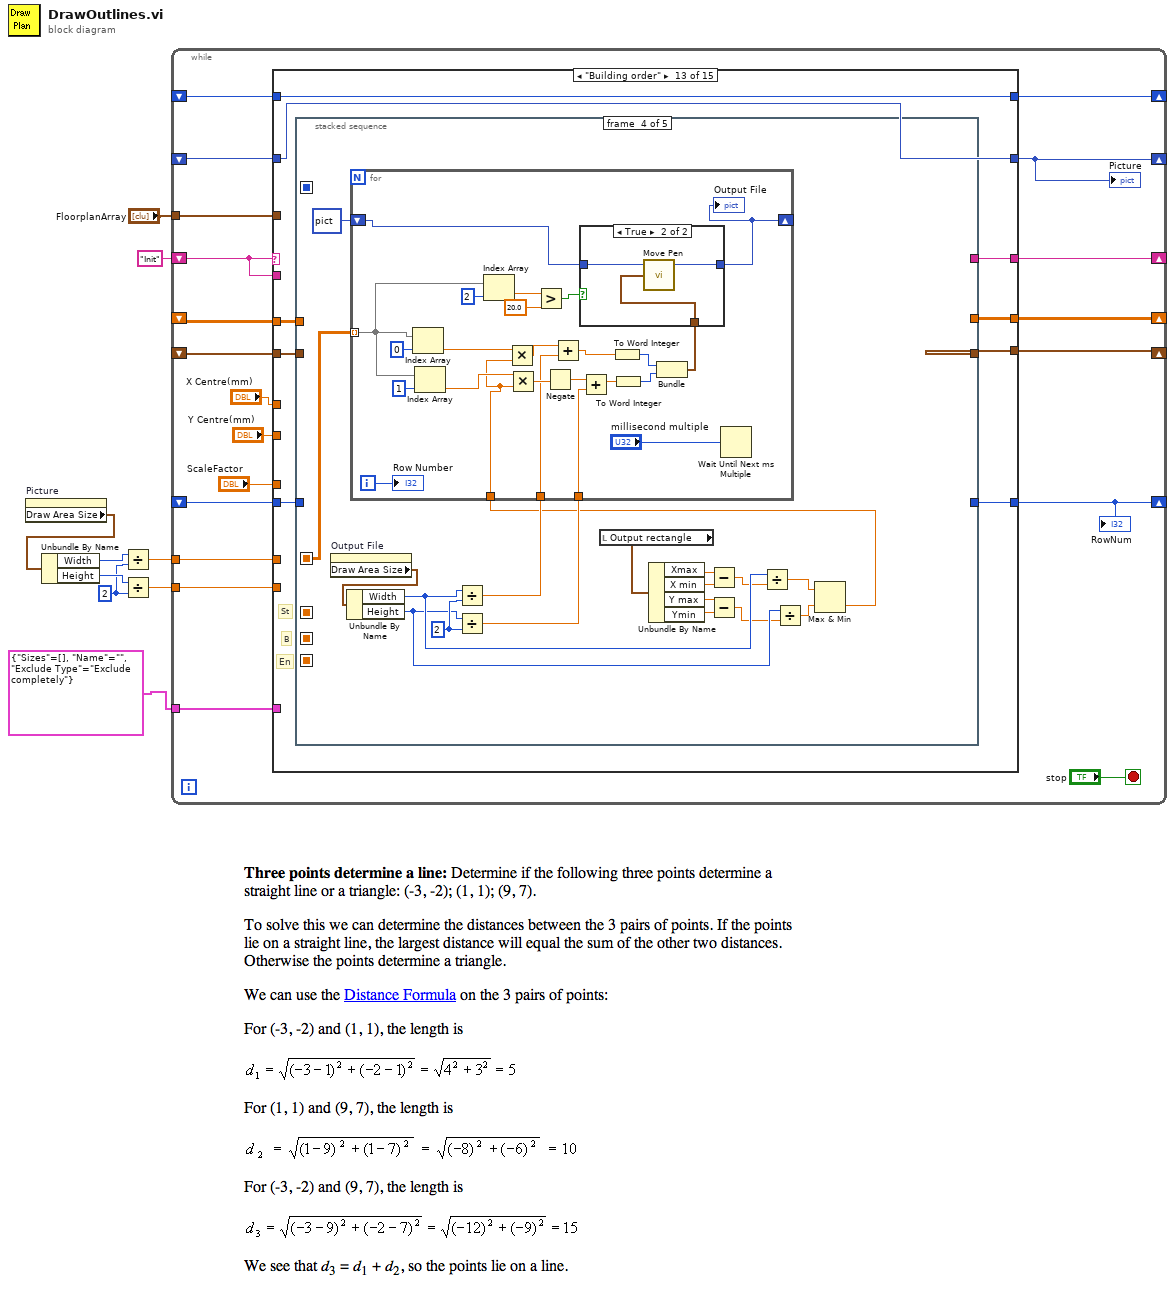
[diagram p0: block diagram]
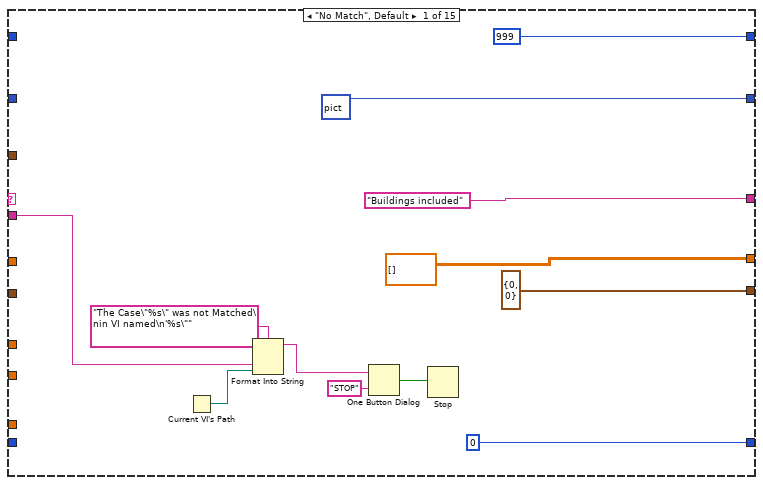
[diagram p2: hidden frame]
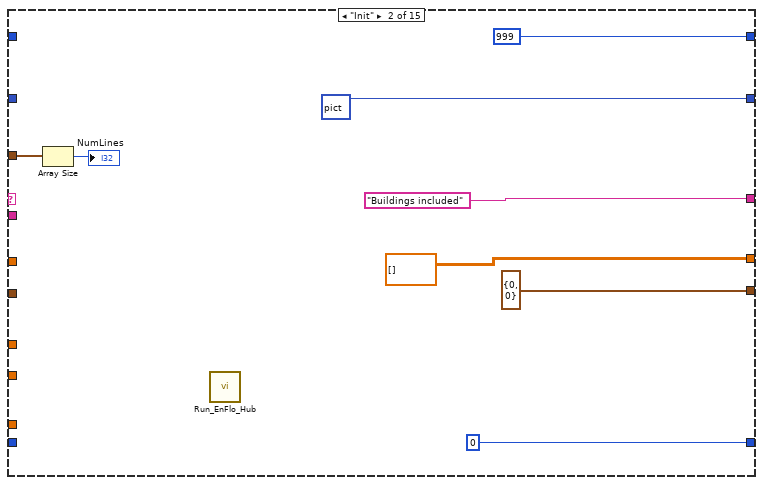
[diagram p3: hidden frame]
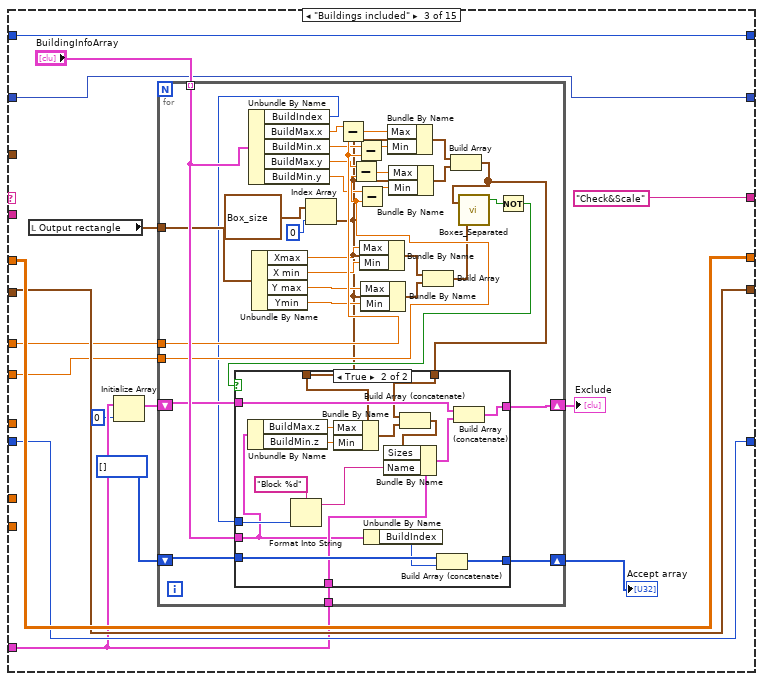
[diagram p4: hidden frame]
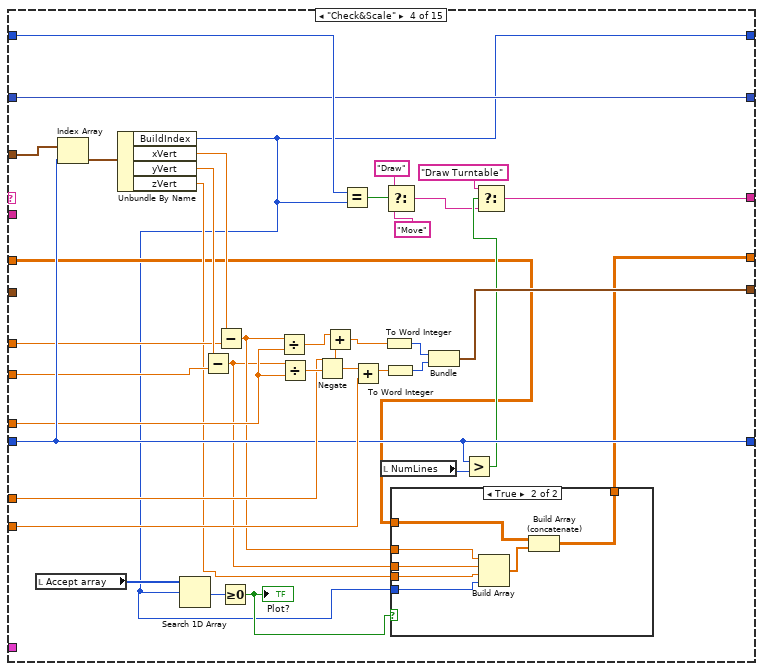
[diagram p6: hidden frame]
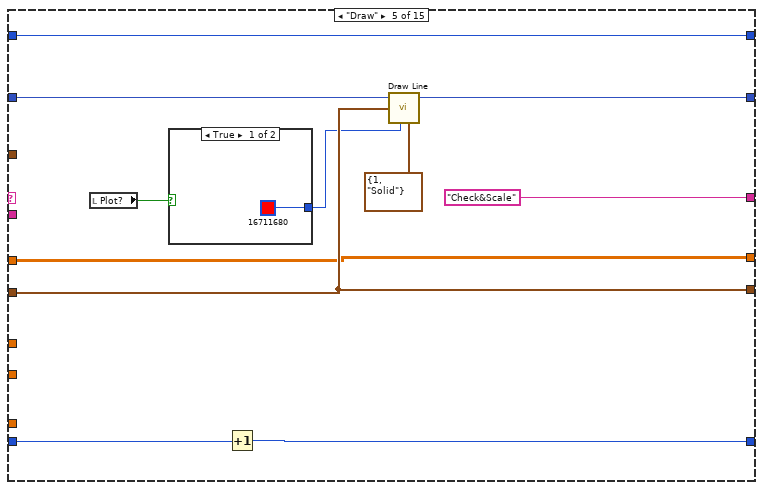
[diagram p8: hidden frame]
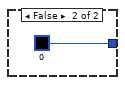
[diagram p9: hidden frame]
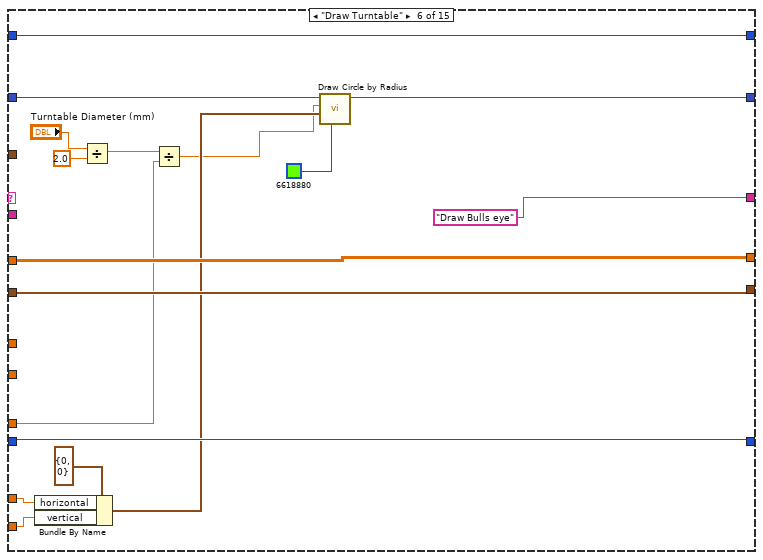
[diagram p10: hidden frame]
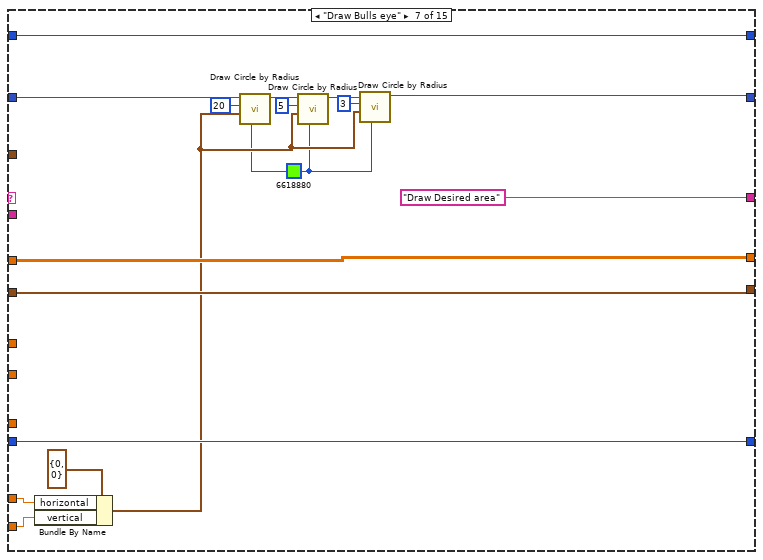
[diagram p11: hidden frame]
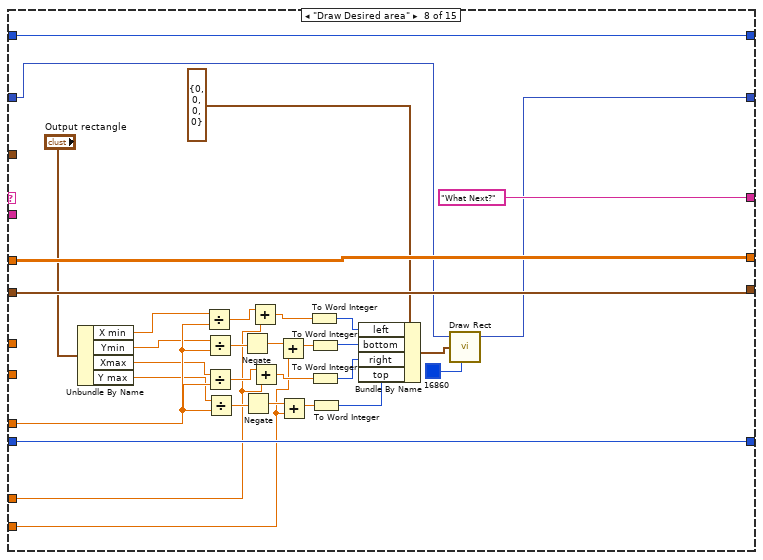
[diagram p12: hidden frame]
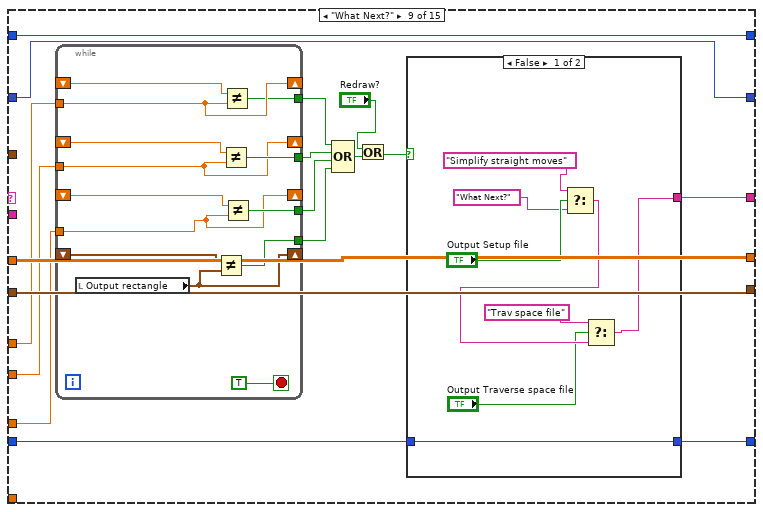
[diagram p13: hidden frame]
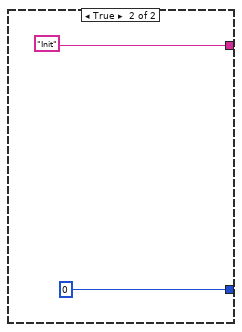
[diagram p14: hidden frame]
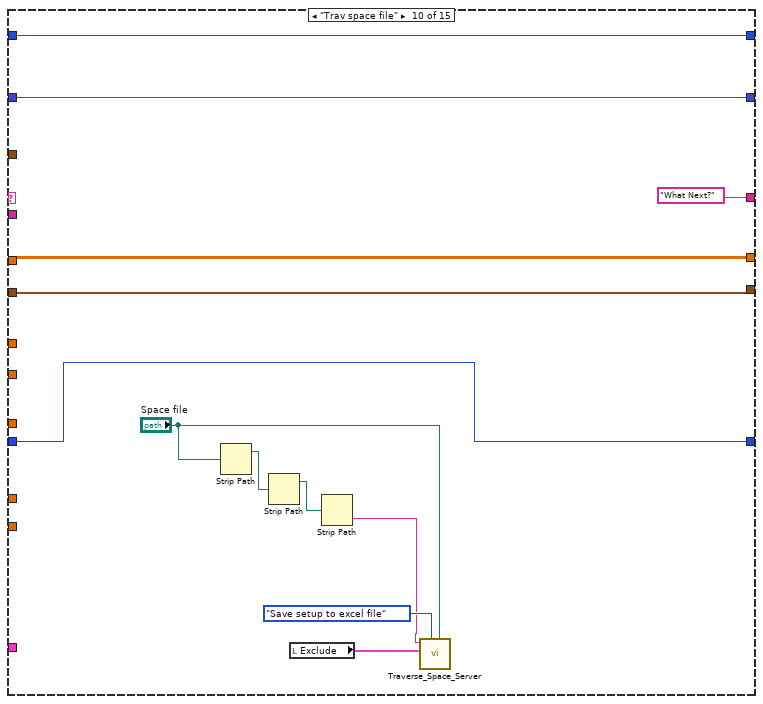
[diagram p15: hidden frame]
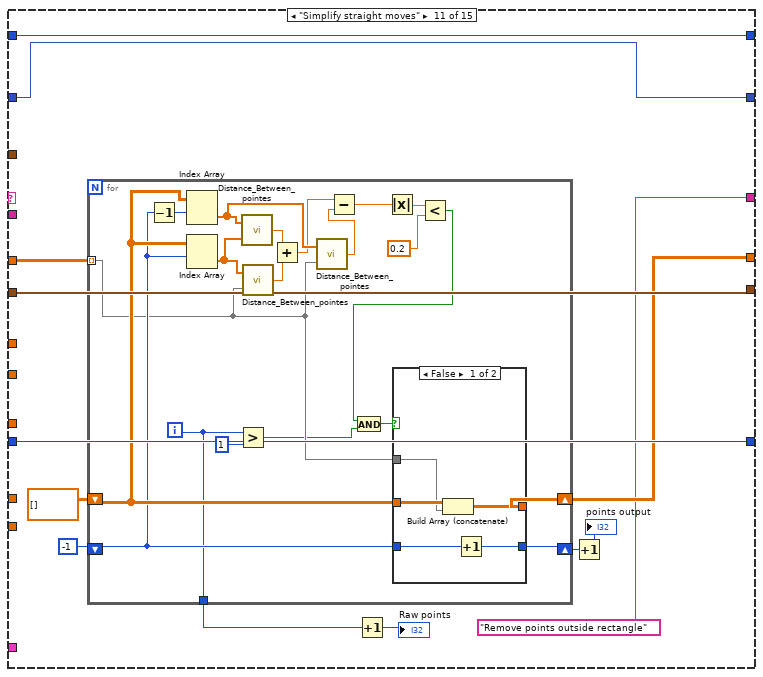
[diagram p16: hidden frame]
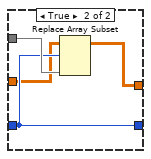
[diagram p17: hidden frame]
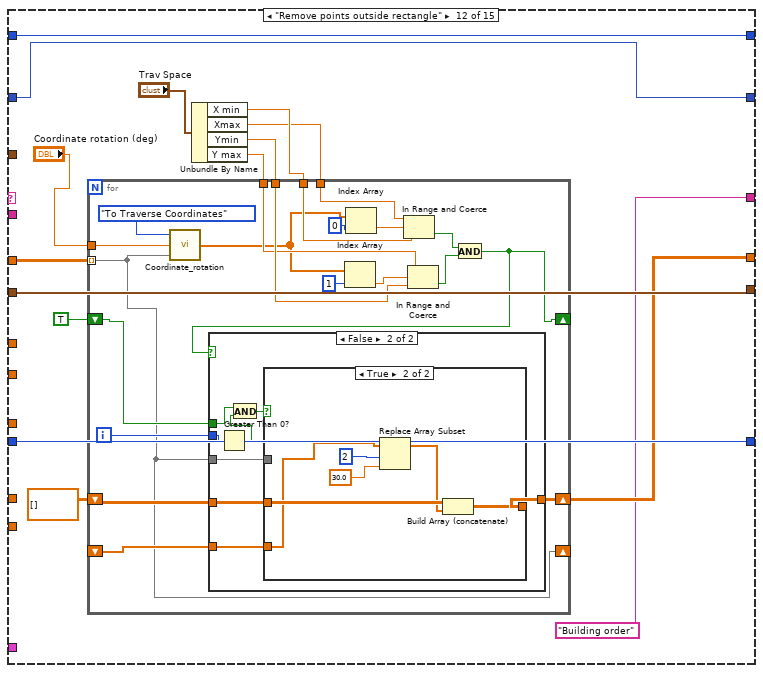
[diagram p18: hidden frame]
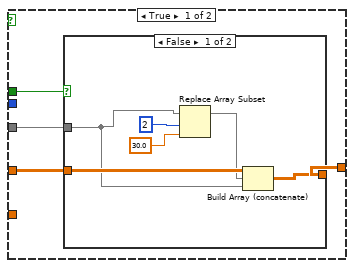
[diagram p19: hidden frame]
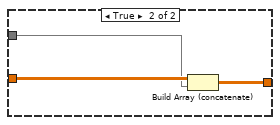
[diagram p20: hidden frame]
diagram:
  w4 = u32 2 ("y")
  n1 = property on="Picture" class="Pict"() -> ("Draw Area Size"=w7:T7)  [unwired: 2 in, 2 out]
  n2 = Unbundle By Name(w7) -> ("Width"=w6:u32, "Height"=w5:u32)
  n3 = Divide(x=w6, y=w4) -> (x/y=w2:dbl)
  n4 = Divide(x=w5, y=w4) -> (x/y=w3:dbl)
  n5 = while {
    shift-right: [w16] -> _
    shift-left: _ -> [w29]
    tunnel: "FloorplanArray" -> [w26]
    shift-right: [w28] -> _
    shift-left: _ -> [w27]
    shift-right: [w17] -> _
    shift-left: "Init" ("f") -> [w12]
    shift-right: [w25] -> _
    shift-left: _ -> [w24]
    shift-right: [w22] -> _
    shift-left: _ -> [w23]
    shift-right: [w21] -> _
    shift-left: _ -> [w20]
    tunnel: w3 -> [w19]
    tunnel: w2 -> [w18]
    tunnel: T1 {"Sizes"=[], "Name"="", "Exclude Type"=enum."Exclude completely"} ("Cluster") -> [w10]
    stop <- "stop" stop-if-true
    n6 = case shown="\"Building order\"" w12 {
      tunnel: [picture data[5B] ("new picture") picture data[5B] ("new picture") w61 w144 w172 w178 w200 w221 w249 w286 w304 w348 w406 w550 w583] -> w16
      tunnel: w29 -> [_ _ w61 w144 w171 w188 w205 w222 w249 w286 w304 w348 w406 w550 w584]
      tunnel: [u32 999 ("BuildIndex") u32 999 ("BuildIndex") w62 w118 w165 w189 w206 w238 w256 w285 w305 w349 w407 w549 w581] -> w28
      tunnel: w27 -> [_ _ w62 w154 w165 w189 w206 w238 w256 w285 w305 w349 w407 w549 w581]
      tunnel: w26 -> [_ w45 _ w150 _ _ _ _ _ _ _ _ _ _ _]
      tunnel: ["Buildings included" ("f") "Buildings included" ("f") "Check&Scale" ("f") w130 "Check&Scale" ("f") "Draw Bulls eye" ("f") "Draw Desired area" ("t") "What Next?" ("t") w252 "What Next?" ("t") "Remove points outside rectangle" ("f") "Building order" ("f") w405 "Init" ("t") "Check&Scale" ("f")] -> w17
      tunnel: [cluster{i16, i16} {0, 0} cluster{i16, i16} {0, 0} w58 w151 w169 w191 w208 w240 w257 w283 w306 w350 w402 w551 w580] -> w25
      tunnel: w24 -> [_ _ w58 _ w169 w191 w208 w240 w257 w283 w306 w350 w401 w551 w580]
      tunnel: [0 ("RowNum") 0 ("RowNum") w57 w133 w167 w190 w207 w239 w251 w282 w303 w347 w400 w552 w578] -> w22
      tunnel: w23 -> [_ _ w57 w133 w168 w190 w207 w239 w250 w282 w303 w347 w399 w552 w579]
      tunnel: [dbl[][] [] dbl[][] [] w59 w119 w166 w192 w209 w241 w258 w284 w299 w344 w403 w546 w577] -> w21
      tunnel: w20 -> [_ _ w59 w120 w166 w192 w209 w241 w258 w284 w302 w346 w404 w546 w577]
      tunnel: w19 -> [_ _ _ w140 _ w186 w203 w216 _ _ _ _ _ _ _]
      tunnel: w18 -> [_ _ _ w139 _ w187 w204 w217 _ _ _ _ _ _ _]
      tunnel: "ScaleFactor" -> [_ _ _ w129 _ w181 _ w226 w246 _ _ _ _ _ _]
      tunnel: "Y Centre(mm)" -> [_ _ w55 w128 _ _ _ _ w247 _ _ _ _ w547 _]
      tunnel: "X Centre(mm)" -> [_ _ w56 w127 _ _ _ _ w248 _ _ _ _ w548 _]
      tunnel: w12 -> [w30 _ _ _ _ _ _ _ _ _ _ _ _ _ _]
      tunnel: w10 -> [_ _ w53 _ _ _ _ _ _ _ _ _ _ _ _]
      frame "No Match", Default {
        n7 = Current VI's Path() -> (path=w31:path)
        n8 = Format Into String(format string="The Case\"%s\" was not Matched\nin VI named\n'%s\"" ("Format String"), w30, w31) -> (resulting string=w34:string)  [unwired: 2 in, 1 out]
        n9 = One Button Dialog(message=w34, button name ("OK")="STOP") -> (true=w32:bool)
        n10 = Stop(stop? (T)=w32) -> ()
      }
      frame "Init" {
        n11 = Array Size(array=w45) -> (size(s)=→"NumLines":i32)
        n12 = call "Run_EnFlo_Hub.vi"() -> ()  [unwired: 8 out]
      }
      frame "Buildings included" {
        n13 = local read "Output rectangle"() -> (w54:T4)
        n14 = Initialize Array(w53, 0 ("dimension size")) -> (w52:T1[])
        n15 = for {
          tunnel: "BuildingInfoArray" -> [w95] mode=indexing
          shift-right: [w96] -> w63
          shift-left: u32[] [] -> [w97]
          tunnel: w56 -> [w94]
          tunnel: w55 -> [w93]
          tunnel: w54 -> [w92]
          shift-right: [w69] -> w50
          shift-left: w52 -> [w70]
          tunnel: w53 -> [w67]
          n16 = Unbundle By Name(w95) -> ("BuildIndex"=w68:u32, "BuildMax.x"=w78:dbl, "BuildMin.x"=w77:dbl, "BuildMax.y"=w75:dbl, "BuildMin.y"=w74:dbl)
          n17 = Unbundle By Name(w92) -> ("Xmax"=w86:dbl, "X min"=w85:dbl, "Y max"=w84:dbl, "Ymin"=w83:dbl)
          n18 = Index Array(array=T2 [{"Max"=16000.0, "Min"=14000.0}, {"Max"=1000.0, "Min"=-1000.0}, {"Max"=700.0, "Min"=0.0}] ("Box 1"), index=0) -> (element=w66:cluster{"Max":dbl, "Min":dbl})
          n19 = Subtract(x=w78, y=w94) -> (x-y=w76:dbl)
          n20 = Subtract(x=w75, y=w93) -> (x-y=w72:dbl)
          n21 = Subtract(x=w77, y=w94) -> (x-y=w79:dbl)
          n22 = Subtract(x=w74, y=w93) -> (x-y=w73:dbl)
          n23 = Bundle By Name(cluster=w66, "Max"=w86, "Min"=w85) -> (w87:cluster{"Max":dbl, "Min":dbl})
          n24 = Bundle By Name(cluster=w66, "Max"=w84, "Min"=w83) -> (w82:cluster{"Max":dbl, "Min":dbl})
          n25 = Bundle By Name(cluster=w66, "Max"=w76, "Min"=w79) -> (w88:cluster{"Max":dbl, "Min":dbl})
          n26 = Bundle By Name(cluster=w66, "Max"=w72, "Min"=w73) -> (w89:cluster{"Max":dbl, "Min":dbl})
          n27 = Build Array(w87, w82) -> (w81:cluster{"Max":dbl, "Min":dbl}[])
          n28 = Build Array(w88, w89) -> (w71:cluster{"Max":dbl, "Min":dbl}[])
          n29 = call "Boxes_Separated.vi"("Box 1"=w71, "Box 2"=w81) -> ("Box Separated"=w80:bool)  [unwired: 2 out]
          n30 = Not(x=w80) -> (.not. x?=w98:bool)
          n31 = case shown="True" w98 {
            tunnel: w97 -> [w100 w117]
            tunnel: [w100 w116] -> w96
            tunnel: w95 -> [_ w105]
            tunnel: w71 -> [_ w104]
            tunnel: w70 -> [w99 w109]
            tunnel: [w99 w108] -> w69
            tunnel: w68 -> [_ w113]
            tunnel: w67 -> [_ w114]
            tunnel: w66 -> [_ w101]
            frame False {
            }
            frame True {
              n32 = Unbundle By Name(w105) -> ("BuildMax.z"=w107:dbl, "BuildMin.z"=w106:dbl)
              n33 = Format Into String(format string="Block %d", w113) -> (resulting string=w112:string)  [unwired: 2 in, 1 out]
              n34 = Bundle By Name(cluster=w101, "Max"=w107, "Min"=w106) -> (w103:cluster{"Max":dbl, "Min":dbl})
              n35 = Unbundle By Name(w105) -> ("BuildIndex"=w115:u32)
              n36 = Build Array (concatenate)(w104, w103) -> (w102:cluster{"Max":dbl, "Min":dbl}[])
              n37 = Bundle By Name(cluster=w114, "Sizes"=w102, "Name"=w112) -> (w110:T1)
              n38 = Build Array (concatenate)(w117, w115) -> (w116:u32[])
              n39 = Build Array (concatenate)(w109, w110) -> (w108:T1[])
            }
          }
        }
        "Accept array" <- w63
        "Exclude" <- w50
      }
      frame "Check&Scale" {
        n40 = local read "Accept array"() -> (w126:u32[])
        n41 = Index Array(array=w150, index=w133) -> (element=w149:T16)
        n42 = Unbundle By Name(w149) -> ("BuildIndex"=w118:u32, "xVert"=w147:dbl, "yVert"=w146:dbl, "zVert"=w121:dbl)
        n43 = Search 1D Array(1D array=w126, element=w118) -> (index of element=w125:i32)  [unwired: 1 out]
        n44 = Subtract(x=w146, y=w128) -> (x-y=w122:dbl)
        n45 = Subtract(x=w147, y=w127) -> (x-y=w123:dbl)
        n46 = Greater Or Equal To 0?(x=w125) -> (x >= 0?=w124:bool)
        "Plot?" <- w124
        n47 = Divide(x=w123, y=w129) -> (x/y=w141:dbl)
        n48 = Divide(x=w122, y=w129) -> (x/y=w142:dbl)
        n49 = Negate(x=w142) -> (-x=w136:dbl)
        n50 = Add(x=w141, y=w139) -> (x+y=w138:dbl)
        n51 = Equal?(x=w154, y=w118) -> (x = y?=w153:bool)
        n52 = Add(x=w136, y=w140) -> (x+y=w137:dbl)
        n53 = local read "NumLines"() -> (w135:i32)
        n54 = To Word Integer(number=w138) -> (16bit integer=w148:i16)
        n55 = To Word Integer(number=w137) -> (16bit integer=w143:i16)
        n56 = Select(t="Draw", s=w153, f="Move") -> (s? t:f=w131:string)
        n57 = case shown="True" w124 {
          tunnel: w123 -> [_ w162]
          tunnel: w122 -> [_ w161]
          tunnel: w121 -> [_ w160]
          tunnel: w120 -> [w155 w158]
          tunnel: [w155 w157] -> w119
          tunnel: w118 -> [_ w156]
          frame False {
          }
          frame True {
            n58 = Build Array(w162, w161, w160, w156) -> (w159:dbl[])
            n59 = Build Array (concatenate)(w158, w159) -> (w157:dbl[][])
          }
        }
        n60 = Bundle(w148, w143) -> (w151:cluster{i16, i16})  [unwired: 1 out]
        n61 = Greater?(x=w133, y=w135) -> (0:w132:bool)
        n62 = Select(t="Draw Turntable", s=w132, f=w131) -> (s? t:f=w130:string)
      }
      frame "Draw" {
        n63 = local read "Plot?"() -> (w163:bool)
        n64 = case shown="True" w163 {
          tunnel: [u32 16711680 ("color(black)") u32 0 ("color(black)")] -> w164
          frame True {
          }
          frame False {
          }
        }
        n65 = Increment(x=w168) -> (x+1=w167:i32)
        n66 = call <vilib>:"Draw Line.vi"("picture"=w171, "end point"=w169, "color(black)"=w164, "pen"=T8 {"Width"=1, "Style"=enum."Solid"}) -> ("new picture"=w172:picture)  [unwired: 1 in, 4 out]
      }
      frame "Draw Turntable" {
        n67 = Bundle By Name(cluster=cluster{"horizontal":i16, "vertical":i16} {"horizontal"=0, "vertical"=0} ("pixel center"), "horizontal"=w187, "vertical"=w186) -> (w185:cluster{"horizontal":i16, "vertical":i16})
        n68 = Divide(x="Turntable Diameter (mm)", y=2.0) -> (x/y=w182:dbl)
        n69 = Divide(x=w182, y=w181) -> (x/y=w180:dbl)
        n70 = call <vilib>:"Draw Circle by Radius.vi"("color(black)"=u32 6618880, "pixel center"=w185, "radius"=w180, "picture"=w188) -> ("new picture"=w178:picture)  [unwired: 4 in, 3 out]
      }
      frame "Draw Bulls eye" {
        w198 = u32 6618880 ("color(black)")
        n71 = Bundle By Name(cluster=cluster{"horizontal":i16, "vertical":i16} {"horizontal"=0, "vertical"=0} ("pixel center"), "horizontal"=w204, "vertical"=w203) -> (w199:cluster{"horizontal":i16, "vertical":i16})
        n72 = call <vilib>:"Draw Circle by Radius.vi"("color(black)"=w198, "pixel center"=w199, "radius"=i16 20, "picture"=w205) -> ("new picture"=w202:picture)  [unwired: 4 in, 3 out]
        n73 = call <vilib>:"Draw Circle by Radius.vi"("color(black)"=w198, "pixel center"=w199, "radius"=i16 5, "picture"=w202) -> ("new picture"=w201:picture)  [unwired: 4 in, 3 out]
        n74 = call <vilib>:"Draw Circle by Radius.vi"("color(black)"=w198, "pixel center"=w199, "radius"=i16 3, "picture"=w201) -> ("new picture"=w200:picture)  [unwired: 4 in, 3 out]
      }
      frame "Draw Desired area" {
        n75 = Unbundle By Name("Output rectangle") -> ("X min"=w215:dbl, "Ymin"=w212:dbl, "Xmax"=w213:dbl, "Y max"=w214:dbl)
        n76 = Divide(x=w215, y=w226) -> (x/y=w235:dbl)
        n77 = Divide(x=w212, y=w226) -> (x/y=w236:dbl)
        n78 = Divide(x=w213, y=w226) -> (x/y=w228:dbl)
        n79 = Divide(x=w214, y=w226) -> (x/y=w227:dbl)
        n80 = Negate(x=w236) -> (-x=w232:dbl)
        n81 = Negate(x=w227) -> (-x=w231:dbl)
        n82 = Add(x=w235, y=w217) -> (x+y=w234:dbl)
        n83 = Add(x=w228, y=w217) -> (x+y=w229:dbl)
        n84 = Add(x=w232, y=w216) -> (x+y=w233:dbl)
        n85 = Add(x=w231, y=w216) -> (x+y=w230:dbl)
        n86 = To Word Integer(number=w234) -> (16bit integer=w219:i16)
        n87 = To Word Integer(number=w233) -> (16bit integer=w211:i16)
        n88 = To Word Integer(number=w229) -> (16bit integer=w218:i16)
        n89 = To Word Integer(number=w230) -> (16bit integer=w210:i16)
        n90 = Bundle By Name(cluster=T9 {"left"=0, "top"=0, "right"=0, "bottom"=0} ("rect"), "left"=w219, "bottom"=w211, "right"=w218, "top"=w210) -> (w223:T9)
        n91 = call <vilib>:"Draw Rect.vi"("picture"=w222, "rect"=w223, "color(black)"=u32 16860) -> ("new picture"=w221:picture)  [unwired: 2 in, 4 out]
      }
      frame "What Next?" {
        n92 = while {
          shift-right: [w280] -> _
          shift-left: _ -> [w281]
          tunnel: w248 -> [w280]
          shift-right: [w273] -> _
          shift-left: _ -> [w279]
          shift-right: [w272] -> _
          shift-left: _ -> [w278]
          tunnel: [w276] -> w255
          tunnel: [w275] -> w254
          tunnel: [w274] -> w253
          tunnel: w247 -> [w273]
          tunnel: w246 -> [w272]
          shift-right: [w270] -> _
          shift-left: _ -> [w271]
          tunnel: [w269] -> w245
          stop <- TRUE stop-if-true
          n93 = local read "Output rectangle"() -> (w270:T4)
          n94 = Not Equal?(x=w271, y=w270) -> (x != y?=w269:bool)
          n95 = Not Equal?(x=w279, y=w273) -> (x != y?=w275:bool)
          n96 = Not Equal?(x=w281, y=w280) -> (x != y?=w276:bool)
          n97 = Not Equal?(x=w278, y=w272) -> (x != y?=w274:bool)
        }
        n98 = Compound Arithmetic op=OR(w255, w254, w253, w245) -> (w244:bool)
        n99 = Or(x="Redraw?", y=w244) -> (x .or. y?=w243:bool)
        n100 = case shown="False" w243 {
          tunnel: [w261 "Init" ("t")] -> w252
          tunnel: [w266 0 ("RowNum")] -> w251
          tunnel: w250 -> [w266 _]
          frame False {
            n101 = Select(t="Simplify straight moves", s="Output Setup file", f="What Next?" ("t")) -> (s? t:f=w262:string)
            n102 = Select(t="Trav space file", s="Output Traverse space file", f=w262) -> (s? t:f=w261:string)
          }
          frame True {
          }
        }
      }
      frame "Trav space file" {
        n103 = Strip Path(path="Space file") -> (stripped path=w291:path)  [unwired: 1 out]
        n104 = Strip Path(path=w291) -> (stripped path=w290:path)  [unwired: 1 out]
        n105 = local read "Exclude"() -> (w293:T1[])
        n106 = Strip Path(path=w290) -> (name=w289:string)  [unwired: 1 out]
        n107 = call "Traverse_Space_Server.vi"("Space File"="Space file", "Mode"=T10."Save setup to excel file", "Exclude Array"=w293, "Traverse Name"=w289) -> ()  [unwired: 3 in, 4 out]
      }
      frame "Simplify straight moves" {
        n108 = for {
          shift-right: [w326] -> w299
          shift-left: dbl[][] [] -> [w323]
          tunnel: w302 -> [w318] mode=indexing
          shift-right: [w325] -> w297
          shift-left: -1 -> [w321]
          tunnel: [w307] -> w294
          i -> [w307]
          n109 = Decrement(x=w321) -> (x-1=w322:i32)
          n110 = Index Array(array=w323, index (row)=w322) -> (element=w319:dbl[])  [unwired: 1 in]
          n111 = Index Array(array=w323, index (row)=w321) -> (element=w320:dbl[])  [unwired: 1 in]
          n112 = Greater?(x=w307, y=1) -> (0:w310:bool)
          n113 = call "Distance_Between_pointes.vi"("P2"=w320, "P1"=w319) -> ("Distance"=w317:dbl)
          n114 = call "Distance_Between_pointes.vi"("P2"=w318, "P1"=w320) -> ("Distance"=w316:dbl)
          n115 = Add(x=w317, y=w316) -> (x+y=w314:dbl)
          n116 = call "Distance_Between_pointes.vi"("P2"=w318, "P1"=w319) -> ("Distance"=w315:dbl)
          n117 = Subtract(x=w314, y=w315) -> (x-y=w313:dbl)
          n118 = Absolute Value(x=w313) -> (abs(x)=w312:dbl)
          n119 = Less?(x=w312, y=0.2) -> (x < y?=w308:bool)
          n120 = And(x=w308, y=w310) -> (x .and. y?=w309:bool)
          n121 = case shown="False" w309 {
            tunnel: w323 -> [w331 w332]
            tunnel: [w330 w334] -> w326
            tunnel: w318 -> [w327 w335]
            tunnel: w321 -> [w329 w333]
            tunnel: [w328 w333] -> w325
            frame False {
              n122 = Build Array (concatenate)(w331, w327) -> (w330:dbl[][])
              n123 = Increment(x=w329) -> (x+1=w328:i32)
            }
            frame True {
              n124 = Replace Array Subset(array=w332, new element=w335, index (row)=w333) -> (w334:dbl[][])  [unwired: 1 in]
            }
          }
        }
        n125 = Increment(x=w294) -> (x+1=→"Raw points":i32)
        n126 = Increment(x=w297) -> (x+1=→"points output":i32)
      }
      frame "Remove points outside rectangle" {
        n127 = Unbundle By Name("Trav Space") -> ("X min"=w342:dbl, "Xmax"=w341:dbl, "Ymin"=w339:dbl, "Y max"=w338:dbl)
        n128 = for {
          shift-right: [w370] -> w344
          shift-left: dbl[][] [] -> [w369]
          tunnel: w346 -> [w355] mode=indexing
          tunnel: w342 -> [w367]
          tunnel: w341 -> [w366]
          tunnel: w339 -> [w364]
          tunnel: w338 -> [w363]
          shift-right: [w360] -> _
          shift-left: TRUE -> [w359]
          shift-right: [w355] -> _
          shift-left: _ -> [w358]
          tunnel: "Coordinate rotation (deg)" -> [w354]
          i -> [w357]
          n129 = call "Coordinate_rotation.vi"("Input Position"=w355, "Coordinate rotation (deg)"=w354, "Mode"=T11."To Traverse Coordinates") -> ("Output Position"=w353:dbl[])
          n130 = Index Array(array=w353, index=1) -> (element=w352:dbl)
          n131 = Index Array(array=w353, index=0) -> (element=w351:dbl)
          n132 = In Range and Coerce(upper limit=w366, x=w351, lower limit=w367) -> (In Range?=w361:bool)  [unwired: 1 out]
          n133 = In Range and Coerce(upper limit=w363, x=w352, lower limit=w364) -> (In Range?=w362:bool)  [unwired: 1 out]
          n134 = And(x=w361, y=w362) -> (x .and. y?=w360:bool)
          n135 = case shown="False" w360 {
            tunnel: [w374 w391] -> w370
            tunnel: w369 -> [w373 w390]
            tunnel: w358 -> [_ w389]
            tunnel: w359 -> [w372 w385]
            tunnel: w355 -> [w371 w388]
            tunnel: w357 -> [_ w387]
            frame True {
              n136 = case shown="False" w372 {
                tunnel: w373 -> [w380 w383]
                tunnel: [w379 w382] -> w374
                tunnel: w371 -> [w378 w381]
                frame False {
                  n137 = Replace Array Subset(array=w378, new element=30.0 ("new element/subarray"), index=2) -> (w375:dbl[])
                  n138 = Build Array (concatenate)(w380, w375, w378) -> (w379:dbl[][])
                }
                frame True {
                  n139 = Build Array (concatenate)(w383, w381) -> (w382:dbl[][])
                }
              }
            }
            frame False {
              n140 = Greater Than 0?(x=w387) -> (x > 0?=w386:bool)
              n141 = And(x=w385, y=w386) -> (x .and. y?=w384:bool)
              n142 = case shown="True" w384 {
                tunnel: w390 -> [w392 w398]
                tunnel: [w392 w397] -> w391
                tunnel: w388 -> [_ _]
                tunnel: w389 -> [_ w393]
                frame False {
                }
                frame True {
                  n143 = Replace Array Subset(array=w393, new element=30.0 ("new element/subarray"), index=2) -> (w394:dbl[])
                  n144 = Build Array (concatenate)(w398, w394) -> (w397:dbl[][])
                }
              }
            }
          }
        }
      }
      frame "Building order" {
        # "B"
        # "En"
        # "St"
        n145 = stacked-sequence {
          seq-local: [w412 _ _ _ _] -> [_ w450 _ _ _]
          seq-local: [w411 _ _ _ _] -> [_ w461 w476 _ _]
          seq-local: [w408 _ _ _ _] -> [_ w453 _ _ _]
          seq-local: [_ w456 _ _ _] -> [_ _ w477 _ _]
          seq-local: [_ _ w473 _ _] -> [_ _ _ w495 _]
          tunnel: [_ _ _ _ "Output Multi run file" ("f")] -> w405
          tunnel: w404 -> [w416 _ w474 _ _]
          tunnel: [_ _ w473 _ _] -> w403
          tunnel: [_ _ _ _ w544] -> w402
          tunnel: w401 -> [_ _ _ _ w544]
          tunnel: [_ _ _ _ w543] -> w400
          tunnel: w399 -> [_ _ _ _ w543]
          frame #0 {
            w414 = dbl[][] []
            # "Bldg"
            # "Start"
            # "End"
            n146 = for {
              tunnel: w416 -> [w422] mode=indexing
              shift-right: [w420] -> _
              shift-left: -100.0 ("Numeric") -> [w428]
              shift-right: [w417] -> w412
              shift-left: w414 -> [w423]
              shift-right: [w418] -> w411
              shift-left: dbl[] [] -> [w419]
              shift-right: [w425] -> w409
              shift-left: w414 -> [w426]
              shift-right: [w422] -> w410
              shift-left: _ -> [w421]
              i -> [w424]
              n147 = Index Array(array=w422, index=3) -> (element=w420:dbl)
              n148 = Equal?(x=w428, y=w420) -> (x = y?=w427:bool)
              n149 = case shown="False" w427 {
                tunnel: w426 -> [w439 w444]
                tunnel: [w433 w444] -> w425
                tunnel: w421 -> [w438 _]
                tunnel: w424 -> [w437 _]
                tunnel: w423 -> [w436 w446]
                tunnel: w422 -> [w435 _]
                tunnel: [w434 w446] -> w417
                tunnel: w420 -> [w431 _]
                tunnel: w419 -> [w432 w445]
                tunnel: [w430 w445] -> w418
                frame False {
                  n150 = case shown="1, Default" w437 {
                    tunnel: w439 -> [w440 w443]
                    tunnel: [w440 w442] -> w433
                    tunnel: w438 -> [_ w441]
                    frame 0 {
                    }
                    frame 1, Default {
                      n151 = Build Array (concatenate)(w443, w441) -> (w442:dbl[][])
                    }
                  }
                  n152 = Build Array (concatenate)(w436, w435) -> (w434:dbl[][])
                  n153 = Build Array (concatenate)(w432, w431) -> (w430:dbl[])
                }
                frame True {
                }
              }
            }
            n154 = Build Array (concatenate)(w409, w410) -> (w408:dbl[][])
          }
          frame #1 {
            n155 = Array Size(array=w461) -> (size(s)=w460:i32)
            n156 = Decrement(x=w460) -> (x-1=w459:i32)
            n157 = Index Array(array=w453, index (row)=0) -> (element=w454:dbl[])  [unwired: 1 in]
            n158 = Initialize Array(10000000.0 ("element"), 4 ("dimension size")) -> (w448:dbl[])
            n159 = Replace Array Subset(array=w450, new element=w448, index (row)=0) -> (w447:dbl[][])  [unwired: 1 in]
            n160 = for {
              N: w459 -> [_]
              tunnel: [w464] -> w457 mode=indexing
              shift-right: [w467] -> _
              shift-left: w447 -> [w468]
              shift-right: [w465] -> _
              shift-left: w454 -> [w466]
              tunnel: w453 -> [w463]
              tunnel: w448 -> [w462]
              n161 = for {
                tunnel: w466 -> [w472]
                tunnel: w468 -> [w471] mode=indexing
                tunnel: [w470] -> w469 mode=indexing
                n162 = call "Distance_Between_pointes.vi"("P2"=w471, "P1"=w472) -> ("Distance"=w470:dbl)
              }
              n163 = Array Max & Min(array=w469) -> (min index (indices)=w464:i32)  [unwired: 3 out]
              n164 = Replace Array Subset(array=w468, new element=w462, index (row)=w464) -> (w467:dbl[][])  [unwired: 1 in]
              n165 = Index Array(array=w463, index (row)=w464) -> (element=w465:dbl[])  [unwired: 1 in]
            }
            n166 = Build Array (concatenate)(0 ("min index(es)"), w457) -> (w456:i32[])
          }
          frame #2 {
            n167 = for {
              tunnel: w477 -> [w483] mode=indexing
              tunnel: w476 -> [w482]
              tunnel: w474 -> [w481]
              shift-right: [w478] -> w473
              shift-left: dbl[][] [] -> [w479]
              n168 = Index Array(array=w482, index=w483) -> (element=w480:dbl)
              n169 = for {
                tunnel: w481 -> [w485] mode=indexing
                tunnel: w480 -> [w488]
                shift-right: [w486] -> w478
                shift-left: w479 -> [w484]
                n170 = Index Array(array=w485, index=3) -> (element=w489:dbl)
                n171 = Equal?(x=w488, y=w489) -> (x = y?=w487:bool)
                n172 = case shown="True" w487 {
                  tunnel: w484 -> [w491 w494]
                  tunnel: [w491 w493] -> w486
                  tunnel: w485 -> [_ w492]
                  frame False {
                  }
                  frame True {
                    n173 = Build Array (concatenate)(w494, w492) -> (w493:dbl[][])
                  }
                }
              }
            }
          }
          frame #3 {
            w512 = u32 2 ("y")
            n174 = property on="Output File" class="Pict"() -> ("Draw Area Size"=w509:T7)  [unwired: 2 in, 2 out]
            n175 = Unbundle By Name(w509) -> ("Width"=w502:u32, "Height"=w500:u32)
            n176 = Divide(x=w502, y=w512) -> (x/y=w511:dbl)
            n177 = Divide(x=w500, y=w512) -> (x/y=w510:dbl)
            n178 = local read "Output rectangle"() -> (w507:T4)
            n179 = Unbundle By Name(w507) -> ("Xmax"=w503:dbl, "X min"=w506:dbl, "Y max"=w505:dbl, "Ymin"=w504:dbl)
            n180 = Subtract(x=w503, y=w506) -> (x-y=w501:dbl)
            n181 = Subtract(x=w505, y=w504) -> (x-y=w499:dbl)
            n182 = Divide(x=w502, y=w501) -> (x/y=w497:dbl)
            n183 = Divide(x=w500, y=w499) -> (x/y=w498:dbl)
            n184 = Max & Min(x=w497, y=w498) -> (min(x,y)=w496:dbl)  [unwired: 1 out]
            n185 = for {
              tunnel: w511 -> [w529]
              tunnel: w510 -> [w528]
              shift-right: [w519] -> _
              shift-left: picture data[5B] ("new picture") -> [w520]
              tunnel: w495 -> [w524] mode=indexing
              tunnel: w496 -> [w517]
              i -> [w513]
              n186 = Index Array(array=w524, index=0) -> (element=w522:dbl)
              n187 = Index Array(array=w524, index=1) -> (element=w523:dbl)
              n188 = Index Array(array=w524, index=2) -> (element=w515:dbl)
              n189 = Multiply(x=w522, y=w517) -> (x*y=w533:dbl)
              n190 = Multiply(x=w523, y=w517) -> (x*y=w534:dbl)
              n191 = Greater?(x=w515, y=20.0) -> (0:w516:bool)
              n192 = Negate(x=w534) -> (-x=w530:dbl)
              n193 = Add(x=w533, y=w529) -> (x+y=w532:dbl)
              n194 = Add(x=w530, y=w528) -> (x+y=w531:dbl)
              n195 = To Word Integer(number=w532) -> (16bit integer=w536:i16)
              n196 = To Word Integer(number=w531) -> (16bit integer=w535:i16)
              n197 = Bundle(w536, w535) -> (w521:cluster{i16, i16})  [unwired: 1 out]
              n198 = case shown="True" w516 {
                tunnel: w521 -> [w537 w542]
                tunnel: w520 -> [w539 w541]
                tunnel: [w538 w540] -> w519
                frame False {
                  n199 = call <vilib>:"Draw Line.vi"("picture"=w539, "end point"=w537) -> ("new picture"=w538:picture)  [unwired: 3 in, 4 out]
                }
                frame True {
                  n200 = call <vilib>:"Move Pen.vi"("new position"=w542, "picture"=w541) -> ("new picture"=w540:picture)  [unwired: 1 in, 2 out]
                }
              }
              "Output File" <- w519
              n201 = Wait Until Next ms Multiple(millisecond multiple="millisecond multiple") -> ()  [unwired: 1 out]
              "Row Number" <- w513
            }
          }
          frame #4 {
          }
        }
      }
      frame "Output Multi run file" {
        w558 = TRUE  # Jump Bad Positions
        n202 = Bundle By Name(cluster=T12 {"Start X"=0.0, "Start Y"=0.0, "Start Z"=0.0, "End X"=0.0, "End Y"=0.0, "End Z"=0.0, "No. of pts."=0, "Spacing"=enum."Linear", "Filename"=path "", "Tunnel Speed"=0.0, "Averaging time (min)"=0.0, "Extra Commands"="", "Specific Arguments"="", "Emission Rate (l/min)"=0.0, "Trace Gas Concentration (%)"=0.0, "Density Ratio"="", "Comments"="", "Row No"=0, "Row Type Selector"=enum."Move Traverse Only", "Completion time"="", "Row Duration (mins)"=0.0, "No. of Valid pts."=0, "Meas Setup File"=""} ("Table-read"), "Row Type Selector"=Multi_run_mode."Move Traverse Only", "Specific Arguments"="No Backlash") -> (w556:T12)
        n203 = for {
          tunnel: w556 -> [w576]
          tunnel: w546 -> [w567] mode=indexing
          tunnel: [w569] -> w555 mode=indexing
          tunnel: w548 -> [w565]
          tunnel: w547 -> [w564]
          n204 = Index Array(array=w567, index=0) -> (element=w572:dbl)
          n205 = Index Array(array=w567, index=1) -> (element=w571:dbl)
          n206 = Index Array(array=w567, index=2) -> (element=w570:dbl)
          n207 = Index Array(array=w567, index=3) -> (element=w563:dbl)
          n208 = Format Into String(format string="Centre X=%.1f Y= %.1f bldg No %d", w565, w564, w563) -> (resulting string=w562:string)  [unwired: 2 in, 1 out]
          n209 = Bundle By Name(cluster=w576, "Start X"=w572, "Start Y"=w571, "Start Z"=w570, "Comments"=w562) -> (w569:T12)
        }
        n210 = call "Save_Trav_setup.vi"("Work in Tunnel Coordinates?"=Tunnel_Coordinates."Work in Model Coordinates", "Trav Table"=w555, "Jump Bad Positions"=w558, "Setup filename"="Setup filename") -> ()  [unwired: 2 out]
      }
      frame "Move" {
        n211 = Increment(x=w579) -> (x+1=w578:i32)
        n212 = call <vilib>:"Move Pen.vi"("new position"=w580, "picture"=w584) -> ("new picture"=w583:picture)  [unwired: 1 in, 2 out]
      }
    }
    "RowNum" <- w22
    "Picture" <- w16
  }
